vi "Text control 2 v1.1.vi"() -> ()   [LabVIEW 2016]
panel:
  in  "Serial Settings:Serial End Mode for Reads":u16(ring)=2 items=["None", "LastBit", "TermChar"]
  in  "Pump No":string="1"
  in  "bytes to read":u32=5
  in  "Timeout (ms)":u32=10000
  in  "Enable Termination\nChar (T)":bool=TRUE
  in  "Termination char\n(0xA = '\\n' = LF)\n(0xD = '\\r' = CR)":u8=13 format="%.0x"
  in  "flow control":u16(ring) items=["None"=0, "XON/XOFF"=1, "RTS/CTS"=2, "DTR/DSR"=4]
  in  "stop bits":u16(ring)=10 items=["1.0"=10, "1.5"=15, "2.0"=20]
  in  "parity":u16(ring) items=["None", "Odd", "Even", "Mark", "Space"]
  in  "data bits":u16=8 min=5 max=8 step=1
  in  "VISA resource name":refnum<visa-resource-name>="COM8"
  in  "baud rate":u32=9600
  out "Serial output":string
  out "error out":errorcluster
  in  "Units":bool
  out "Elapsed Time":dbl caption="Elapsed Time (s)"
  out "Ion vs time":cluster{"Y data in":dbl[], "X data in":dbl[]}[](graph)
  out "Ig":dbl format="%.2e"
  out "Id":dbl format="%.2e"
  out "Is":dbl format="%.2e"
  out "I vs Vg":cluster{"Y data in":dbl[], "X data in":dbl[]}[](graph)
  in  "Panel Controls 2":T1={"Emergency Stop"=refnum, "TransGraph Max"=1e-05, "Text/Graph (text=false)"=TRUE, "TransGraph Min"=1e-11} {"TransGraph Min" format="%.2e"; "TransGraph Max" format="%.2e"}
  out "Currently running:":string="#output s 0 0 0 -0.008 0.008 0.002"
  in  "Lines left to run:":string
  in  "Standby":T2
  in  "Full Reset":bool
  in  "SMU4":cluster{"on/off":bool, "Voltage":dbl} {"Voltage" min=-100.0 max=100.0 format="%.2f"}
  in  "Source/Drain Range":u8(slide)=6 max=11 scale=0.0..11.0
  in  "Source/Drain\nRange mode":u16(ring) items=["Auto", "Limited", "Fixed"]
  in  "Gate Range":u8(slide)=6 max=11 scale=0.0..11.0
  in  "Gate Range\nmode":u16(ring) items=["Auto", "Limited", "Fixed"]
  in  "Gate":T3={"Gate Start"=0.0, "Gate Stop"=2.0, "Gate Step (linear only)"=1.0, "Gate Compliance"=0.0001, "Gate PComp"=0.0, "Range mode"=0, "Range"=6} {"Range" max=11 scale=0.0..11.0; "Range mode" items=["Auto", "Limited", "Fixed"]; "Gate PComp" format="%^.2e"; "Gate Compliance" format="%^.2e"; "Gate Step (linear only)" format="%^.4e"; "Gate Stop" format="%^.4e"; "Gate Start" format="%^.4e"}
  in  "Drain 2":T4={"Drain Start"=0.0, "Drain Stop"=2.0, "Drain Compliance"=0.0001, "Drain Step"=1.0, "Drain PComp"=0.0, "Range mode"=0, "Range"=6} {"Range" max=11 scale=0.0..11.0; "Range mode" items=["Auto", "Limited", "Fixed"]; "Drain PComp" format="%^.2e"; "Drain Step" format="%^.4e"; "Drain Compliance" format="%^.2e"; "Drain Stop" format="%^.4e"; "Drain Start" format="%^.4e"}
  in  "Timings 2":T5={"integration time"=0, "Short/Long integration time"=0.00064, "hold time (sec)"=0.0, "delay time (sec)"=0.0, "Step Time (0 disables)"=0.0, "sweep method"=0, "Pulse period"=0.005, "Base voltage"=0.0, "Pulse width"=0.0005} {"Pulse width" min=0.0005 max=0.1 step=0.0001 format="%.4f"; "Base voltage" format="%^.4e"; "Pulse period" min=0.005 max=1.0 step=0.0001 format="%.4f"; "sweep method" items=["Continuous", "Pulsed"]; "Step Time (0 disables)" format="%.2f"; "delay time (sec)" format="%.4f"; "hold time (sec)" format="%.4f"; "Short/Long integration time" format="%^.0e"; "integration time" scale=0.0..2.0}
  in  "Panel Controls":T6={"Emergency Stop"=refnum, "TransGraph Max"=1e-05, "Text/Graph (text=false)"=TRUE} {"TransGraph Max" format="%.2e"}
  in  "Interrupt run":bool
  in  "Drain: Compliance":dbl=0.001 format="%.8f"
  in  "Gate: Compliance":dbl=0.001 format="%.8f"
  out "Path":path=path "C:/users/rlp38/09Apr2009LTtesting/test2.txt"
  in  "hold time /s":dbl format="%.2f"
  in  "delay time /s":dbl format="%.2f"
  in  "integration time":u32(slide) max=2 step=1 scale=0.0..2.0
  in  "Integration time (short)":dbl=0.0019 min=8e-05 max=0.0019 step=8e-05 format="%^.0e"
  in  "Integration time (long)":dbl=0.32 min=0.04 max=2.0 step=0.02 format="%.2f"
  in  "Step delay /s":dbl format="%.2f"
  in  "Program":string="#pulsedstressV d 0.03 20 0 0.5 0.0827 5\n#\n#itime s\n#gaterangemode l\n#drainrangemode l\n#pulsed on 0.05 0 0.02\n#transfer d 1 -1 -0.1 -1 -1 0\n#wait-min 1\n#transfer d 1 -1 -0.1 -1 -1 0\n#output d 0 -1 -0.5 0 -1 -0.1\n#transfer d -10 40 1 5 40 35\n#transfer d -10 40 1 5 40 35\n#output d 0 40 20 0 40 1\n#\n#\n#sample 1 0.008 221 6 0.003\n#samplei 400e-6 200 6 0.002 0.1\n#vsu2pulse -10 4\n#\n#stressV 0.016 0.03 2e-4 0.1e-3 11\n#stressI 220e-7 0.08 15\n#transfer s -1 1 0.5 -0.005 0.005 0.005\n#output s 0 0 0 -0.008 0.008 0.002\n"
  # "Syntax:\nitime [s|m|l]\ngaterangemode [a|l|f]\ndrainrangemode [a|l|f]\npulsed [on|off] PulsePeriod(sec) PulseBaseVoltage PulseONWidth(sec)\nstandby [on l off]\nwait NumMilliseconds\nwait-min NumMinutes\n# texthere = comment\ntransfer [s|d] VgStart VgStop VgStep VdStart VdStop VdStep\noutput [s|d] VgStart VgStop VgStep VdStart VdStop VdStep\nsample Vg Vd NumSamples Time(s) SampleInterval(s)\nsamplei Idg NumSamples Time(s) SampleInterval(s) VDGcompliance\n# if in doubt use SampleInterval(s) = 0.004\nstressV VG VD IGcompliance IDcompliance Duration(sec)\nstressI IDG VDGcompliance Duration(sec)\nvsu2pulse Bias Duration(s)\npulsedstressV [s|d] VEstop VgON VgOFF Period(s) PulseONwidth(s) Vd\nsample-fpp Vg Vd NumSamples Time\nresample-fpp Vg Vd\ntransfer-fpp [s|d] VgStart VgStop VgStep VdStart VdStop VdStep\noutput-fpp [s|d] VgStart VgStop VgStep VdStart VdStop VdStep"
  # "Time"
  # "Sec"
  # "Min"
  # "100 samples is approx 13s with medium integration"
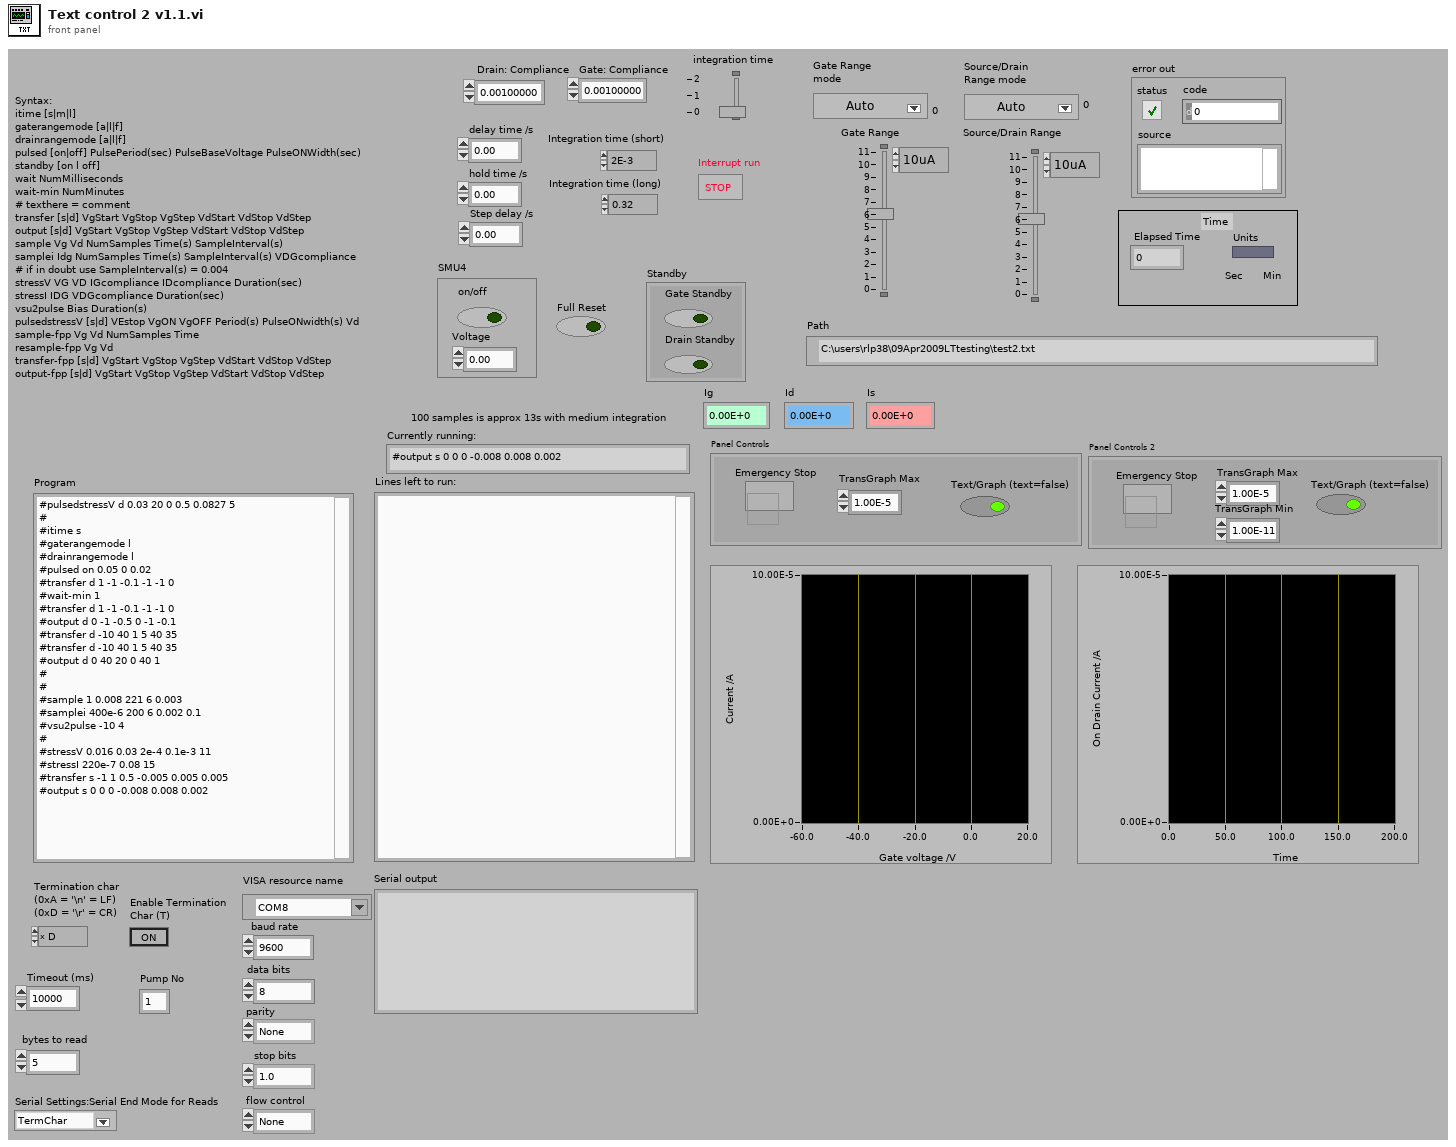
[diagram p1: front panel]
types:
  T1 = cluster{"Emergency Stop":refnum<vi>, "TransGraph Max":dbl, "Text/Graph (text=false)":bool, "TransGraph Min":dbl}
  T2 = cluster{"Gate Standby":bool, "Drain Standby":bool}
  T3 = cluster{"Gate Start":dbl, "Gate Stop":dbl, "Gate Step (linear only)":dbl, "Gate Compliance":dbl, "Gate PComp":dbl, "Range mode":u16, "Range":u8}
  T4 = cluster{"Drain Start":dbl, "Drain Stop":dbl, "Drain Compliance":dbl, "Drain Step":dbl, "Drain PComp":dbl, "Range mode":u16, "Range":u8}
  T5 = cluster{"integration time":u32, "Short/Long integration time":dbl, "hold time (sec)":dbl, "delay time (sec)":dbl, "Step Time (0 disables)":dbl, "sweep method":u16, "Pulse period":dbl, "Base voltage":dbl, "Pulse width":dbl}
  T6 = cluster{"Emergency Stop":refnum<vi>, "TransGraph Max":dbl, "Text/Graph (text=false)":bool}
  T7 = enum16{"open", "replace", "create", "open or create", "replace or create", "replace or create with confirmation"}
  T8 = cluster{"V2 Start":dbl, "V2 Step":dbl, "Number of points":i32}
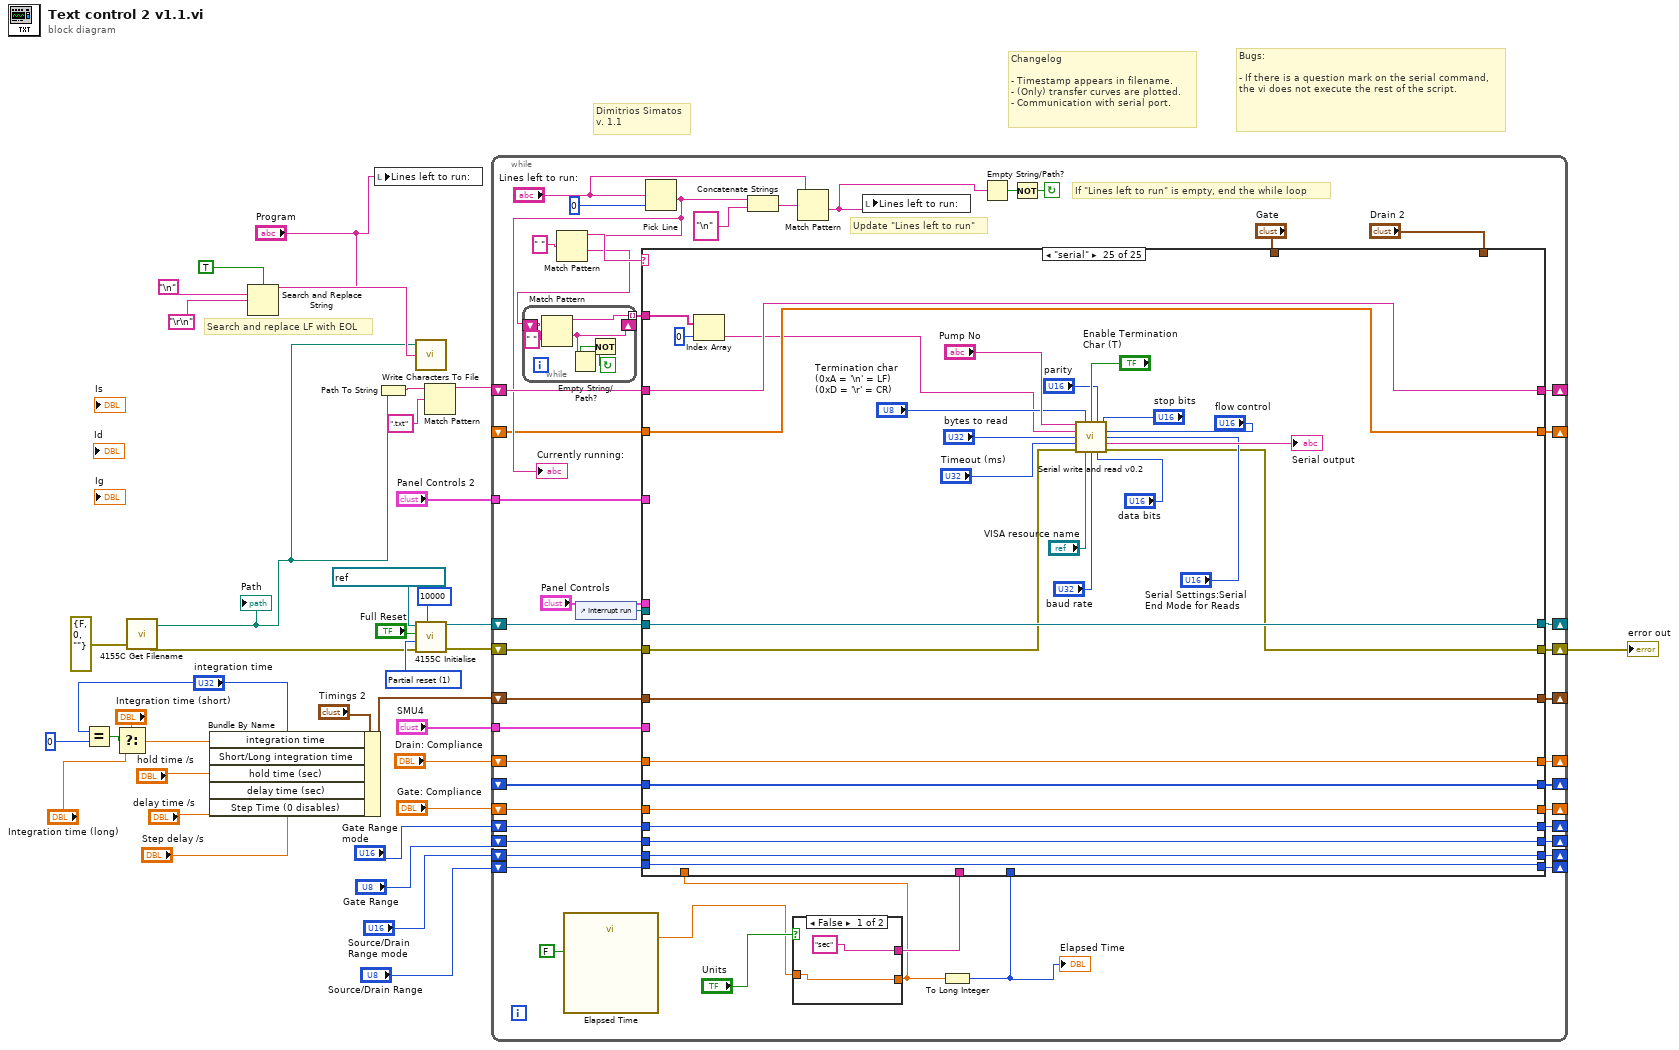
[diagram p0: block diagram]
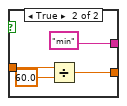
[diagram p2: hidden frame]
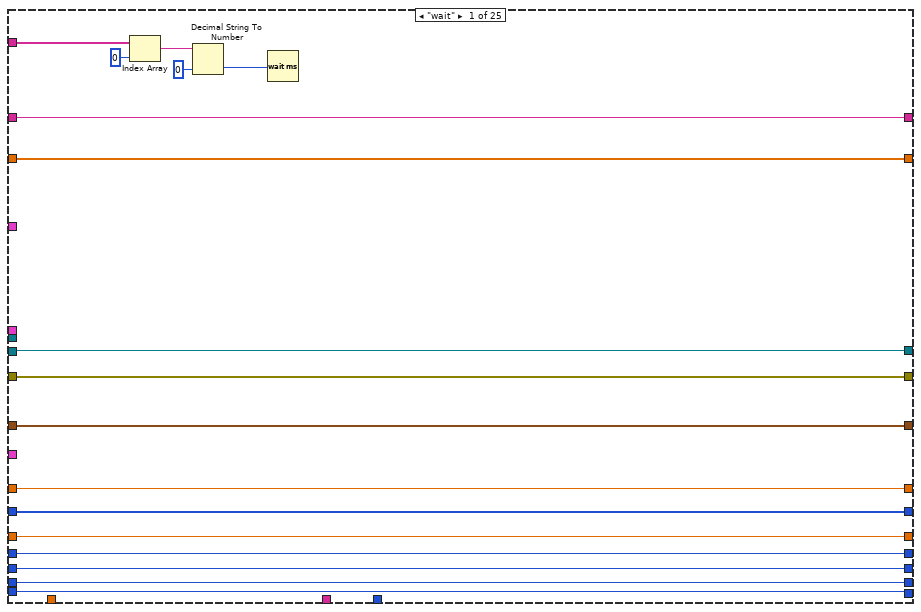
[diagram p3: hidden frame]
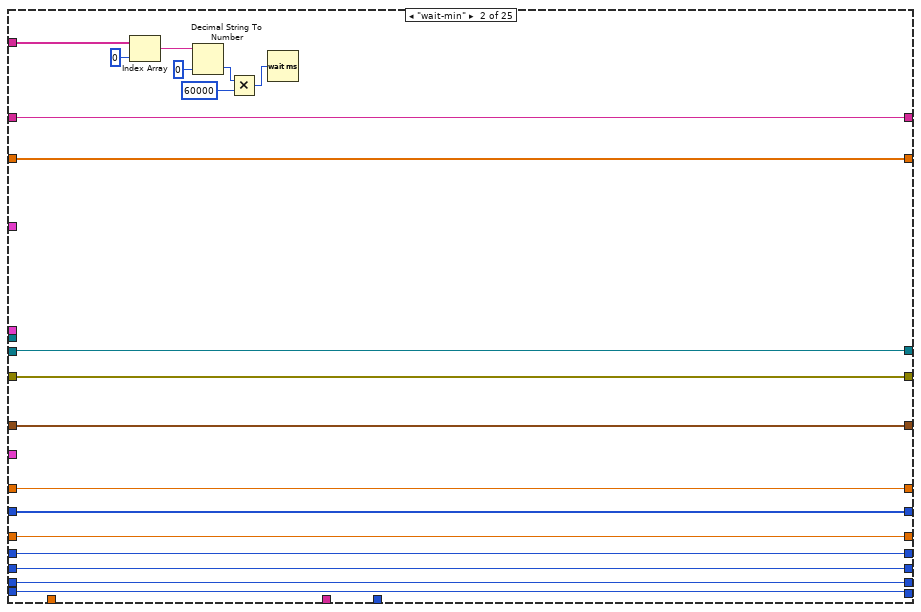
[diagram p4: hidden frame]
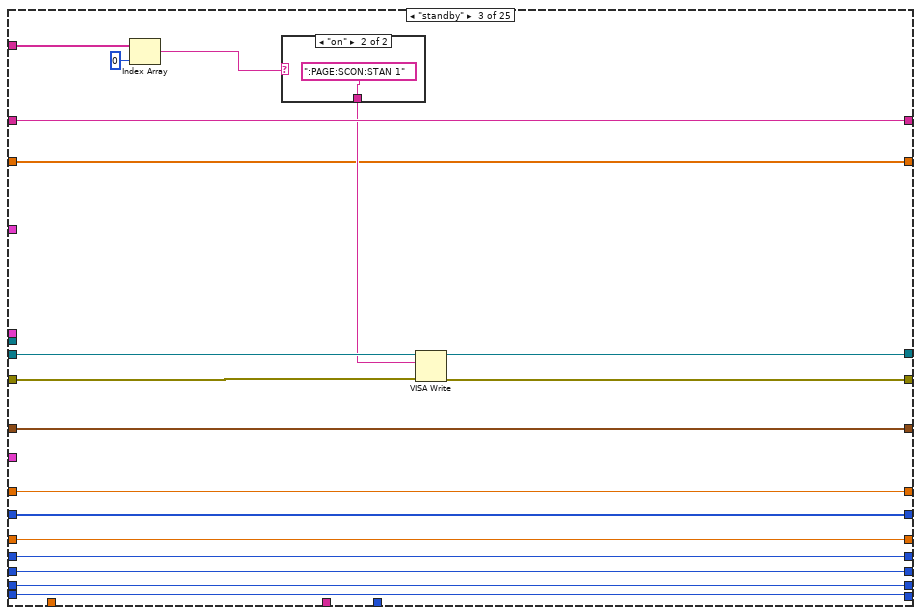
[diagram p5: hidden frame]
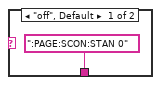
[diagram p6: hidden frame]
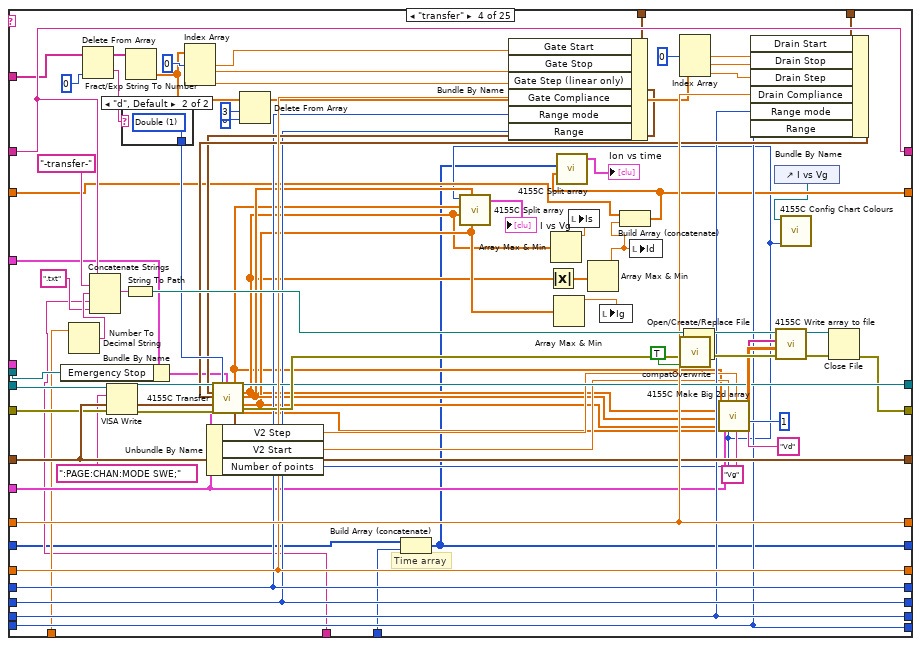
[diagram p7: hidden frame]
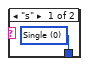
[diagram p8: hidden frame]
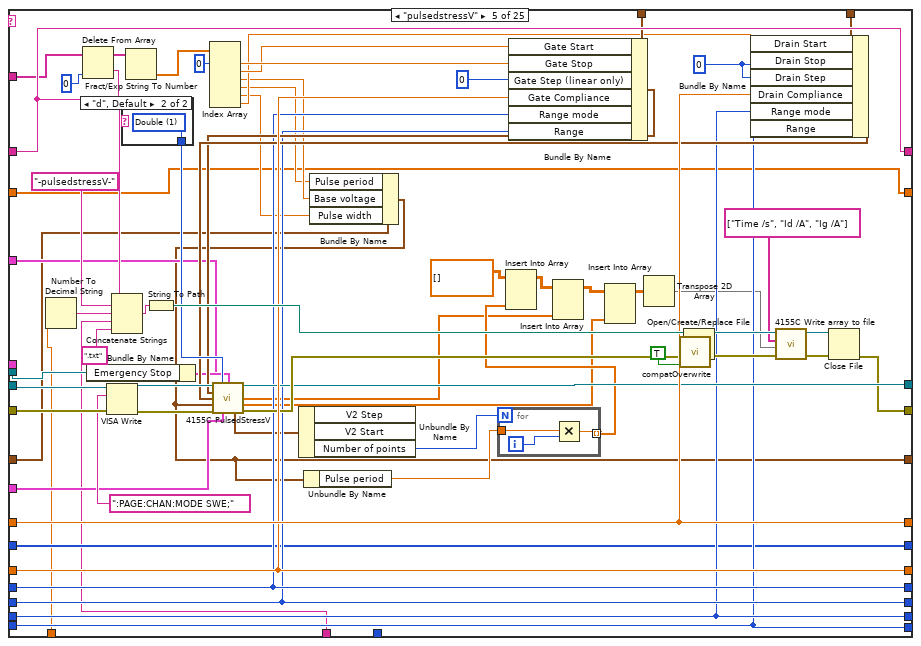
[diagram p9: hidden frame]
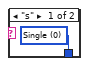
[diagram p10: hidden frame]
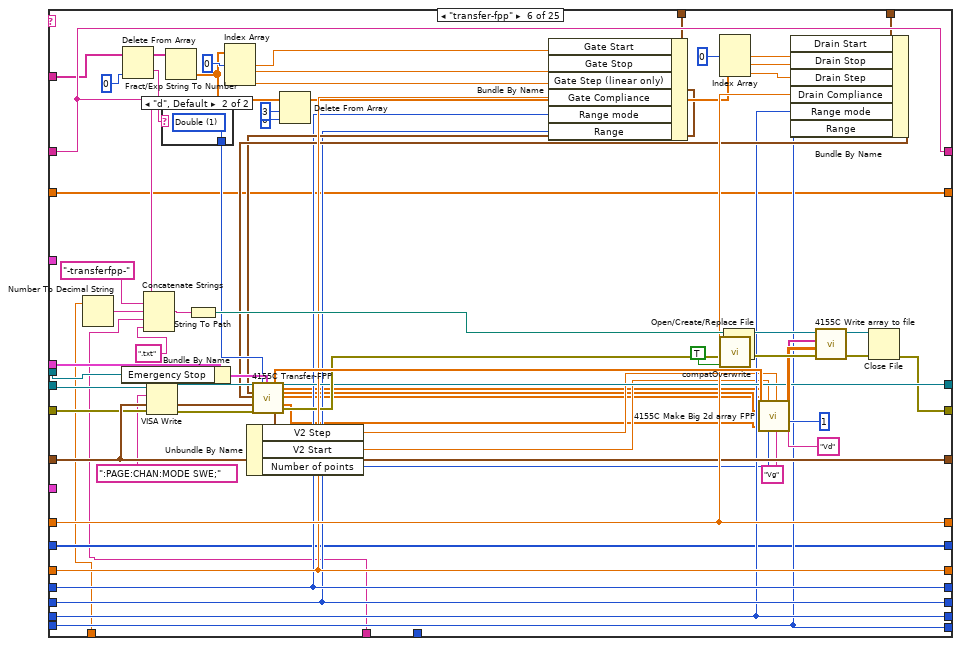
[diagram p11: hidden frame]
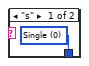
[diagram p12: hidden frame]
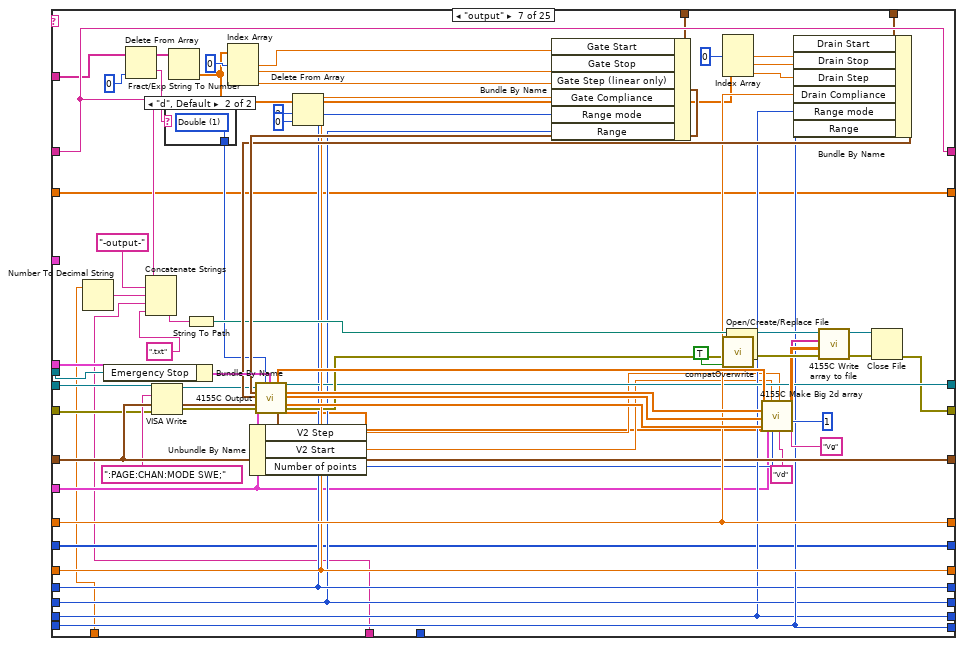
[diagram p13: hidden frame]
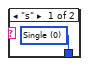
[diagram p14: hidden frame]
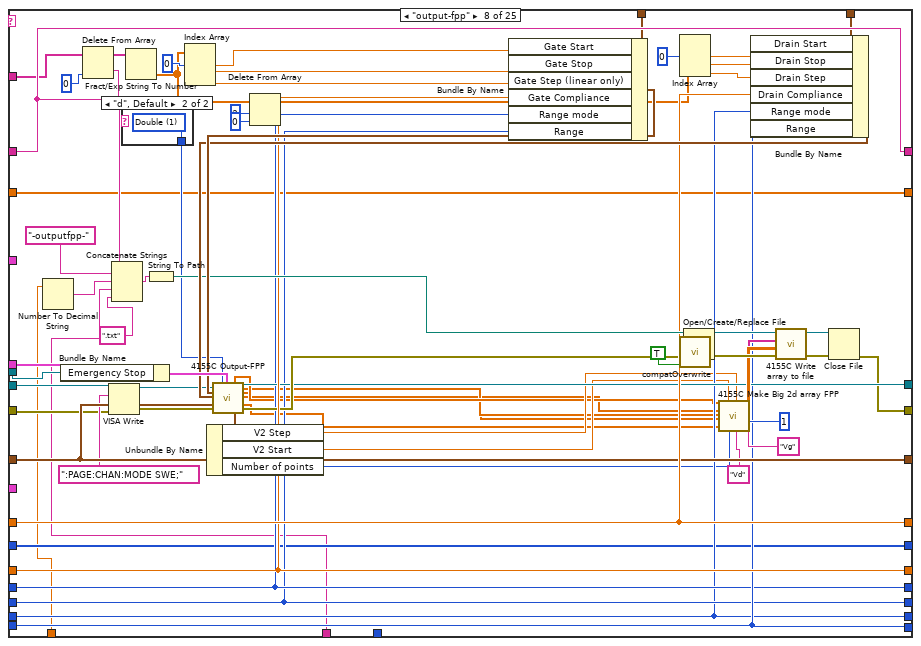
[diagram p15: hidden frame]
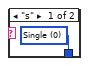
[diagram p16: hidden frame]
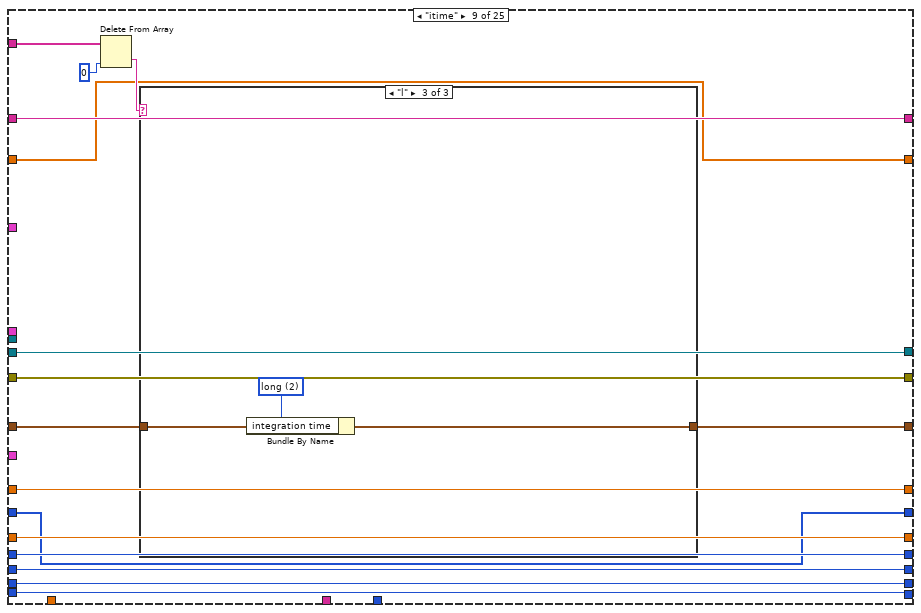
[diagram p17: hidden frame]
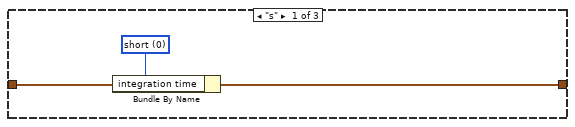
[diagram p18: hidden frame]
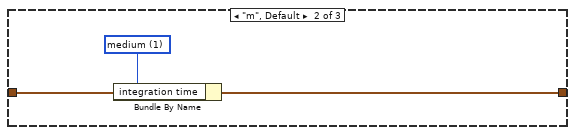
[diagram p19: hidden frame]
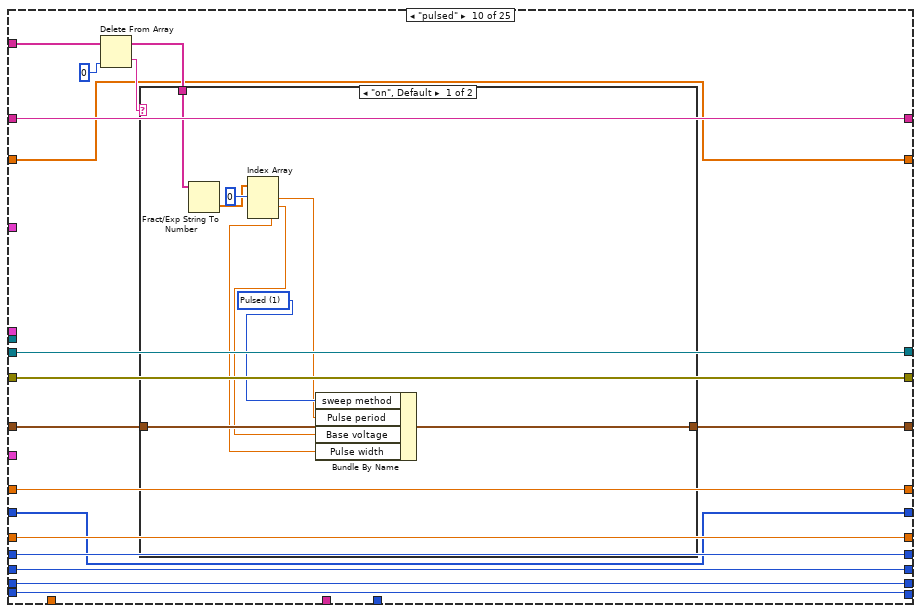
[diagram p20: hidden frame]
diagram:
  w28 = u16 1 items=["Reset All", "Partial reset"] ("Type of reset")
  # "Search and replace LF with EOL"
  # "Bugs:\n\n- If there is a question mark on the serial command, the vi does not execute the rest of the script."
  # "Dimitrios Simatos\nv. 1.1"
  # "Changelog\n\n- Timestamp appears in filename.\n- (Only) transfer curves are plotted.\n- Communication with serial port."
  n1 = Equal?(x="integration time", y=u32 0) -> (x = y?=w32:bool)
  n2 = Select(t="Integration time (short)", s=w32, f="Integration time (long)") -> (s? t:f=w36:dbl)
  n3 = call <userlib>:"4155C Get Filename.vi"("error in (no error)"=errorcluster {"status"=FALSE, "code"=0, "source"=""}) -> ("error out"=w23:errorcluster, "path"=w7:path)  [unwired: 2 in, 1 out]
  "Path" <- w7
  n4 = Bundle By Name(cluster="Timings 2", "integration time"="integration time", "Short/Long integration time"=w36, "hold time (sec)"="hold time /s", "delay time (sec)"="delay time /s", "Step Time (0 disables)"="Step delay /s") -> (w20:T5)
  n5 = Search and Replace String(replace all?=TRUE ("replace all? (F)"), input string="Program", search string="\n", replace string="\r\n") -> (result string=w10:string)  [unwired: 4 in, 3 out]
  n6 = local write "Lines left to run:"("Program") -> ()
  n7 = Path To String(path=w7) -> (string=w6:string)
  n8 = call <vilib>:"Write Characters To File.vi"("character string"=w10, "file path (dialog if empty)"=w7) -> ()  [unwired: 3 in, 1 out]
  n9 = call <userlib>:"4155C Initialise.vi"("VISA resource name in"=refnum<visa-resource-name> "GPIB0::14::INSTR", "Reset"="Full Reset", "Type of reset"=w28, "error in (no error)"=w23, "VISA Timeout Value"=u32 10000) -> ("VISA Resource Name out"=w22:refnum<visa-resource-name>, "error out"=w21:errorcluster)
  n10 = Match Pattern(string=w6, regular expression=".txt") -> (before substring=w5:string)  [unwired: 1 in, 3 out]
  n11 = while {
    tunnel: "SMU4" -> [w52]
    shift-left: "Source/Drain Range" -> [w57]
    shift-right: [w53] -> _
    shift-left: "Source/Drain\nRange mode" -> [w58]
    shift-right: [w54] -> _
    shift-left: "Gate Range" -> [w59]
    shift-right: [w55] -> _
    shift-left: "Gate Range\nmode" -> [w60]
    shift-right: [w56] -> _
    shift-left: "Gate: Compliance" -> [w71]
    shift-right: [w66] -> _
    shift-left: "Drain: Compliance" -> [w72]
    shift-right: [w67] -> _
    shift-left: w20 -> [w73]
    shift-right: [w68] -> _
    shift-left: w21 -> [w74]
    shift-right: [w69] -> w2
    shift-left: w22 -> [w75]
    shift-right: [w70] -> _
    shift-left: w5 -> [w76]
    shift-right: [w65] -> _
    tunnel: "Panel Controls 2" -> [w48]
    shift-right: [w47] -> _
    shift-left: _ -> [w46]
    shift-right: [w41] -> _
    shift-left: _ -> [w40]
    stop <- w84 continue-if-true
    # "If \"Lines left to run\" is empty, end the while loop"
    # "Update \"Lines left to run\""
    n12 = call "Elapsed Time"("Auto Reset"=FALSE) -> ("Elapsed Time (s)"=w42:dbl)  [unwired: 11 in, 7 out]
    n13 = control-ref of="Interrupt run"() -> (w64:refnum<vi>)
    n14 = Pick Line(multi-line string="Lines left to run:", line index=0) -> (output string=w49:string)  [unwired: 1 in]
    "Currently running:" <- w49
    n15 = Match Pattern(string=w49, regular expression=" ") -> (before substring=w79:string, after substring=w78:string)  [unwired: 1 in, 2 out]
    n16 = while {
      tunnel: [w92] -> w77 mode=indexing
      shift-left: w78 -> [w94]
      shift-right: [w93] -> _
      stop <- w96 continue-if-true
      n17 = Match Pattern(string=w94, regular expression=" ") -> (before substring=w92:string, after substring=w93:string)  [unwired: 1 in, 2 out]
      n18 = Empty String/Path?(string/path=w93) -> (empty?=w97:bool)
      n19 = Not(x=w97) -> (.not. x?=w96:bool)
    }
    n20 = Concatenate Strings(w49, "\n" ("Substring")) -> (w82:string)
    n21 = case shown="False" "Units" {
      tunnel: ["sec" "min"] -> w43
      tunnel: [w86 w90] -> w39
      tunnel: w42 -> [w86 w89]
      frame False {
      }
      frame True {
        n22 = Divide(x=w89, y=60.0) -> (x/y=w90:dbl)
      }
    }
    n23 = Match Pattern(string="Lines left to run:", regular expression=w82) -> (after substring=w50:string)  [unwired: 1 in, 3 out]
    n24 = local write "Lines left to run:"(w50) -> ()
    n25 = To Long Integer(number=w39) -> (32bit integer=w38:i32)
    "Elapsed Time" <- w38
    n26 = case shown="\"serial\"" w79 {
      tunnel: w77 -> [w114 w133 w151 w215 w286 w355 w422 w497 w535 w561 w588 w613 w634 w648 _ _ w752 w813 _ w878 w922 w964 w1034 w1096 w1102]
      tunnel: w76 -> [w109 w129 w149 w223 w293 w363 w430 w505 w524 w550 w580 w606 w628 w641 w660 w702 w730 w795 w826 w865 w909 w952 w1028 w1092 w1104]
      tunnel: w75 -> [w108 w128 w140 w193 w277 w332 w398 w473 w525 w551 w581 w607 w629 w642 w665 w704 w758 w819 w830 w884 w928 w970 w1040 w1050 w1108]
      tunnel: w74 -> [w107 w127 w139 w192 w276 w331 w395 w470 w526 w552 w582 w608 w630 w643 w664 w675 w757 w818 w829 w883 w927 w969 w1039 w1049 w1107]
      tunnel: w73 -> [w106 w126 w148 w219 w252 w359 w426 w501 w534 w560 w579 w605 w627 w640 w663 w699 w721 w787 w835 w858 w902 w945 w1027 w1091 w1109]
      tunnel: w72 -> [w105 w125 w147 w221 w291 w361 w428 w503 w533 w559 w587 w612 w633 w647 w662 w684 w756 w817 w838 w882 w926 w968 w1038 w1100 w1110]
      tunnel: w71 -> [w104 w124 w146 w220 w290 w360 w427 w502 w532 w558 w586 w611 w632 w646 w661 w685 w731 w796 w837 w866 w910 w953 w1029 w1093 w1112]
      tunnel: [w108 w128 w138 w217 w288 w357 w424 w499 w525 w551 w581 w607 w629 w642 w665 w704 w722 w769 w828 w859 w903 w946 w980 w1052 w1108] -> w70
      tunnel: [w107 w127 w137 w216 w287 w356 w423 w498 w526 w552 w582 w608 w630 w643 w664 w674 w732 w770 w827 w867 w911 w954 w979 w1051 w1106] -> w69
      tunnel: [w106 w126 w148 w219 w248 w359 w426 w501 w527 w553 w579 w605 w627 w640 w663 w699 w721 w787 w835 w858 w902 w945 w1027 w1091 w1109] -> w68
      tunnel: [w105 w125 w147 w221 w291 w361 w428 w503 w533 w559 w587 w612 w633 w647 w662 w684 w756 w817 w838 w882 w926 w968 w1038 w1100 w1110] -> w67
      tunnel: [w104 w124 w146 w220 w290 w360 w427 w502 w532 w558 w586 w611 w632 w646 w661 w685 w731 w796 w837 w866 w910 w953 w1029 w1093 w1112] -> w66
      tunnel: [w109 w129 w149 w223 w293 w363 w430 w505 w524 w550 w580 w606 w628 w641 w660 w702 w730 w795 w826 w865 w909 w952 w1028 w1092 w1104] -> w65
      tunnel: w64 -> [_ _ _ w226 w297 w368 w438 w509 _ _ _ _ _ _ _ _ w727 w792 _ w864 w908 w951 w1000 w1068 _]
      tunnel: "Gate" -> [_ _ _ w202 w280 w342 w409 w484 _ _ _ _ _ _ _ _ _ _ _ _ _ _ _ _ _]
      tunnel: "Drain 2" -> [_ _ _ w201 w279 w341 w408 w483 _ _ _ _ _ _ _ _ _ _ _ _ _ _ _ _ _]
      tunnel: "Panel Controls" -> [_ _ _ _ _ w340 w407 w482 _ _ _ _ _ _ _ _ _ _ _ _ _ _ _ _ _]
      tunnel: w60 -> [w103 w123 w145 w186 w270 w325 w393 w468 w531 w557 _ w604 w626 w639 w659 w686 w717 w783 w831 w854 w898 w941 w1023 w1087 w1113]
      tunnel: w59 -> [w102 w122 w144 w185 w269 w324 w392 w467 w530 w556 w585 _ w617 w645 w658 w687 w718 w784 w832 w855 w899 w942 w1024 w1088 w1114]
      tunnel: w58 -> [w101 w121 w143 w184 w268 w323 w391 w466 w529 w555 w584 w610 w631 _ w657 w688 w719 w785 w833 w856 w900 w943 w1025 w1089 w1115]
      tunnel: w57 -> [w100 w120 w142 w183 w267 w322 w394 w469 w528 w554 w583 w609 _ w644 w656 w689 w720 w786 w834 w857 w901 w944 w1026 w1090 w1116]
      tunnel: [w103 w123 w145 w186 w270 w325 w393 w468 w531 w557 w578 w604 w626 w639 w659 w686 w717 w783 w831 w854 w898 w941 w1023 w1087 w1113] -> w56
      tunnel: [w102 w122 w144 w185 w269 w324 w392 w467 w530 w556 w585 w596 w617 w645 w658 w687 w718 w784 w832 w855 w899 w942 w1024 w1088 w1114] -> w55
      tunnel: [w101 w121 w143 w184 w268 w323 w391 w466 w529 w555 w584 w610 w631 w638 w657 w688 w719 w785 w833 w856 w900 w943 w1025 w1089 w1115] -> w54
      tunnel: [w100 w120 w142 w183 w267 w322 w394 w469 w528 w554 w583 w609 w618 w644 w656 w689 w720 w786 w834 w857 w901 w944 w1026 w1090 w1116] -> w53
      tunnel: w52 -> [_ _ _ w178 w264 _ w386 _ _ _ _ _ _ _ _ _ _ _ _ _ _ _ _ _ _]
      tunnel: w48 -> [_ _ _ w176 w263 _ _ _ _ _ _ _ _ _ _ _ _ _ _ _ _ _ _ _ _]
      tunnel: [w99 w116 w135 w165 w240 w312 w383 w455 w523 w548 w577 w595 w616 w637 w655 w670 w709 w767 w825 w843 w891 w935 w977 w1045 w1105] -> w47
      tunnel: w46 -> [w99 w116 w135 w164 w240 w312 w383 w455 w523 w548 w577 w595 w616 w637 w655 w670 w709 w767 w825 w843 w891 w935 w977 w1045 w1105]
      tunnel: w39 -> [_ _ _ w160 w237 w310 w380 w452 _ _ _ _ _ _ _ w668 w707 w764 _ w840 w888 w932 w974 w1041 _]
      tunnel: w43 -> [_ _ _ w157 w236 w308 w379 w451 _ _ _ _ _ _ _ w666 w705 w763 _ w839 w887 w931 w973 w1042 _]
      tunnel: w38 -> [_ _ _ w154 _ _ _ _ _ _ _ _ _ _ _ _ _ _ _ _ _ _ _ _ _]
      tunnel: [w98 w115 w134 w156 w239 w311 w382 w454 w522 w547 w576 w594 w615 w636 w654 w669 w708 w766 w824 w842 w890 w934 w976 w1044 w1111] -> w41
      tunnel: w40 -> [w98 w115 w134 w155 w239 w311 w382 w454 w522 w547 w576 w594 w615 w636 w654 w669 w708 w766 w824 w842 w890 w934 w976 w1044 w1111]
      frame "wait" {
        n27 = Index Array(array=w114, index=0 ("Index")) -> (element=w112:string)
        n28 = Decimal String To Number(string=w112, default (0L)=u32 0) -> (number=w111:u32)  [unwired: 1 in, 1 out]
        n29 = Wait (ms)(milliseconds to wait=w111) -> ()  [unwired: 1 out]
      }
      frame "wait-min" {
        n30 = Index Array(array=w133, index=0 ("Index")) -> (element=w131:string)
        n31 = Decimal String To Number(string=w131, default (0L)=u32 0) -> (number=w119:u32)  [unwired: 1 in, 1 out]
        n32 = Multiply(x=w119, y=u32 60000) -> (x*y=w118:u32)
        n33 = Wait (ms)(milliseconds to wait=w118) -> ()  [unwired: 1 out]
      }
      frame "standby" {
        n34 = Index Array(array=w151, index=0 ("Index")) -> (element=w141:string)
        n35 = case shown="\"on\"" w141 {
          tunnel: [":PAGE:SCON:STAN 0" ":PAGE:SCON:STAN 1"] -> w136
          frame "off", Default {
          }
          frame "on" {
          }
        }
        n36 = VISA Write(VISA resource name=w140, write buffer=w136, error in (no error)=w139) -> (VISA resource name out=w138:refnum<visa-resource-name>, error out=w137:errorcluster)  [unwired: 1 out]
      }
      frame "transfer" {
        # "Time array"
        n37 = Bundle By Name(cluster=w176, "Emergency Stop"=w226) -> (w177:T1)
        n38 = Number To Decimal String(number=w160) -> (decimal integer string=w159:string)  [unwired: 1 in]
        n39 = Delete From Array(array=w215, index=0 ("Index")) -> (deleted portion=w213:string, array with subset deleted=w212:string[])  [unwired: 1 in]
        n40 = Concatenate Strings(w223, "-transfer-" ("Prefix"), w159, w157, ".txt" ("Suffix")) -> (w225:string)
        n41 = VISA Write(VISA resource name=w193, write buffer=":PAGE:CHAN:MODE SWE;" ("write buffer (\"\")"), error in (no error)=w192) -> (VISA resource name out=w190:refnum<visa-resource-name>, error out=w191:errorcluster)  [unwired: 1 out]
        n42 = case shown="\"d\", Default" w213 {
          tunnel: [w234 w235] -> w211
          frame "s" {
            w234 = u16 0 items=["Single", "Double"] ("sweep mode")
          }
          frame "d", Default {
            w235 = u16 1 items=["Single", "Double"] ("sweep mode")
          }
        }
        n43 = String To Path(string=w225) -> (path=w222:path)
        n44 = Fract/Exp String To Number(string=w212) -> (number=w197:dbl[])  [unwired: 3 in, 1 out]
        n45 = Index Array(array=w197, index #1=0 ("Index")) -> (element #1=w210:dbl, element #2=w209:dbl, element #3=w208:dbl)  [unwired: 2 in]
        n46 = Delete From Array(array=w197, length=3 ("Length"), index=0 ("Index")) -> (array with subset deleted=w195:dbl[])  [unwired: 1 out]
        n47 = Build Array (concatenate)(w155, w154) -> (w156:i32[])
        n48 = Bundle By Name(cluster=w202, "Gate Start"=w210, "Gate Stop"=w209, "Gate Step (linear only)"=w208, "Gate Compliance"=w220, "Range mode"=w186, "Range"=w185) -> (w187:T3)
        n49 = Index Array(array=w195, index #1=0 ("Index")) -> (element #1=w205:dbl, element #2=w204:dbl, element #3=w203:dbl)  [unwired: 2 in]
        n50 = call <vilib>:"compatOverwrite.vi"("overwrite (F)"=TRUE) -> ("overwrite?"=w175:T7)
        n51 = Bundle By Name(cluster=w201, "Drain Start"=w205, "Drain Stop"=w204, "Drain Step"=w203, "Drain Compliance"=w221, "Range mode"=w184, "Range"=w183) -> (w188:T4)
        n52 = call <userlib>:"4155C Transfer.vi"("VISA resource name in"=w190, "Gate"=w187, "Drain"=w188, "Timings"=w219, "error in (no error)"=w191, "SMU4"=w178, "sweep mode"=w211, "Panel Controls"=w177) -> ("VG"=w166:dbl[], "Outparams"=w182:T8, "VISA Resource Name out"=w217:refnum<visa-resource-name>, "IS"=w168:dbl[], "ID"=w173:dbl[], "IG"=w169:dbl[], "error out"=w218:errorcluster, "SMU4"=w179:dbl[])  [unwired: 12 in]
        n53 = Unbundle By Name(w182) -> ("V2 Step"=w181:dbl, "V2 Start"=w180:dbl, "Number of points"=w162:i32)
        n54 = call <userlib>:"4155C Split array.vi"("Number of VAR2 steps"=w162, "Y2 data in"=w173, "X data in"=w166, "Y1 data in"=w168, "Y3 data in"=w169) -> ("Array of clusters"=→"I vs Vg":cluster{"Y data in":dbl[], "X data in":dbl[]}[])  [unwired: 2 in, 1 out]
        n55 = Absolute Value(x=w168) -> (abs(x)=w172:dbl[])
        n56 = Array Max & Min(array=w168) -> (max value=w170:dbl)  [unwired: 3 out]
        n57 = Array Max & Min(array=w169) -> (max value=w171:dbl)  [unwired: 3 out]
        n58 = local write "Is"(w170) -> ()
        n59 = Array Max & Min(array=w172) -> (max value=w163:dbl)  [unwired: 3 out]
        n60 = local write "Ig"(w171) -> ()
        n61 = Build Array (concatenate)(w164, w163) -> (w165:dbl[])
        n62 = call <userlib>:"4155C Split array.vi"("X data in"=w156, "Y1 data in"=w165) -> ("Array of clusters"=→"Ion vs time":cluster{"Y data in":dbl[], "X data in":dbl[]}[])  [unwired: 5 in, 1 out]
        n63 = local write "Id"(w163) -> ()
        n64 = Open/Create/Replace File(file path (use dialog)=w222, error in=w218, operation (0:open)=w175) -> (refnum out=w231:refnum<file>, error out=w232:errorcluster)  [unwired: 3 in, 1 out]
        n65 = call <userlib>:"4155C Make Big 2d array.vi"("1D Var1"=w166, "1d IS"=w168, "1d ID"=w173, "1d IG"=w169, "1d SMU4"=w179, "SMU4"=w178, "VAR2 START"=w180, "Number of VAR2 steps"=w162, "VAR2 STEP"=w181, "VAR1 Name"="Vg", "Decimal places in header"=i8 1, "VAR2 Name"="Vd") -> ("Header array"=w227:string[], "Data array"=w228:dbl[][])  [unwired: 14 in]
        n66 = control-ref of="I vs Vg"() -> (w161:refnum<vi>)
        n67 = call <userlib>:"4155C Write array to file.vi"("Byte Stream File Refnum"=w231, "Header"=w227, "Data Array"=w228, "error in (no error)"=w232) -> ("dup refnum"=w229:refnum<file>, "error out"=w230:errorcluster)  [unwired: 1 in]
        n68 = call <userlib>:"4155C Config Chart Colours.vi"("Numeric"=w162, "XY Graph 2"=w161) -> ()  [unwired: 6 in]
        n69 = Close File(refnum=w229, error in=w230) -> (error out=w216:errorcluster)  [unwired: 1 out]
      }
      frame "pulsedstressV" {
        w246 = 0
        n70 = Number To Decimal String(number=w237) -> (decimal integer string=w294:string)  [unwired: 1 in]
        n71 = Delete From Array(array=w286, index=0 ("Index")) -> (deleted portion=w284:string, array with subset deleted=w283:string[])  [unwired: 1 in]
        n72 = Bundle By Name(cluster=w263, "Emergency Stop"=w297) -> (w265:T1)
        n73 = VISA Write(VISA resource name=w277, write buffer=":PAGE:CHAN:MODE SWE;" ("write buffer (\"\")"), error in (no error)=w276) -> (VISA resource name out=w274:refnum<visa-resource-name>, error out=w275:errorcluster)  [unwired: 1 out]
        n74 = Concatenate Strings(w293, "-pulsedstressV-" ("Substring"), w294, w236, ".txt" ("Substring")) -> (w296:string)
        n75 = case shown="\"d\", Default" w284 {
          tunnel: [w306 w307] -> w282
          frame "s" {
            w306 = u16 0 items=["Single", "Double"] ("sweep mode")
          }
          frame "d", Default {
            w307 = u16 1 items=["Single", "Double"] ("sweep mode")
          }
        }
        n76 = Fract/Exp String To Number(string=w283) -> (number=w278:dbl[])  [unwired: 3 in, 1 out]
        n77 = String To Path(string=w296) -> (path=w292:path)
        n78 = Index Array(array=w278, index #1=0 ("Index")) -> (element #1=w255:dbl, element #2=w254:dbl, element #3=w251:dbl, element #4=w250:dbl, element #5=w249:dbl, element #6=w253:dbl)  [unwired: 5 in]
        n79 = Bundle By Name(cluster=w252, "Pulse period"=w250, "Base voltage"=w251, "Pulse width"=w249) -> (w248:T5)
        n80 = Unbundle By Name(w248) -> ("Pulse period"=w256:dbl)
        n81 = Bundle By Name(cluster=w280, "Gate Start"=w254, "Gate Stop"=w255, "Gate Step (linear only)"=0, "Gate Compliance"=w290, "Range mode"=w270, "Range"=w269) -> (w271:T3)
        n82 = call <vilib>:"compatOverwrite.vi"("overwrite (F)"=TRUE) -> ("overwrite?"=w241:T7)
        n83 = Bundle By Name(cluster=w279, "Drain Start"=w253, "Drain Stop"=w246, "Drain Step"=w246, "Drain Compliance"=w291, "Range mode"=w268, "Range"=w267) -> (w272:T4)
        n84 = call <userlib>:"4155C PulsedStressV.vi"("VISA resource name in"=w274, "sweep mode"=w282, "Panel Controls"=w265, "Gate"=w271, "Drain"=w272, "Timings"=w248, "error in (no error)"=w275, "SMU4"=w264) -> ("VISA Resource Name out"=w288:refnum<visa-resource-name>, "ID"=w244:dbl[], "IG"=w242:dbl[], "Outparams"=w266:T8, "error out"=w289:errorcluster)  [unwired: 3 in]
        n85 = Unbundle By Name(w266) -> ("Number of points"=w243:i32)  [unwired: 2 out]
        n86 = for {
          N: w243 -> [_]
          tunnel: [w303] -> w245 mode=indexing
          tunnel: w256 -> [w305]
          i -> [w304]
          n87 = Multiply(x=w305, y=w304) -> (x*y=w303:dbl)
        }
        n88 = Insert Into Array(array=dbl[][] [] ("Input Array"), new element=w245) -> (w257:dbl[][])  [unwired: 2 in]
        n89 = Insert Into Array(array=w257, new element=w244) -> (w262:dbl[][])  [unwired: 2 in]
        n90 = Insert Into Array(array=w262, new element=w242) -> (w261:dbl[][])  [unwired: 2 in]
        n91 = Transpose 2D Array(2D array=w261) -> (transposed array=w260:dbl[][])
        n92 = Open/Create/Replace File(file path (use dialog)=w292, error in=w289, operation (0:open)=w241) -> (refnum out=w300:refnum<file>, error out=w301:errorcluster)  [unwired: 3 in, 1 out]
        n93 = call <userlib>:"4155C Write array to file.vi"("Byte Stream File Refnum"=w300, "Header"=string[] ["Time /s", "Id /A", "Ig /A"], "Data Array"=w260, "error in (no error)"=w301) -> ("dup refnum"=w298:refnum<file>, "error out"=w299:errorcluster)  [unwired: 1 in]
        n94 = Close File(refnum=w298, error in=w299) -> (error out=w287:errorcluster)  [unwired: 1 out]
      }
      frame "transfer-fpp" {
        n95 = Number To Decimal String(number=w310) -> (decimal integer string=w364:string)  [unwired: 1 in]
        n96 = Bundle By Name(cluster=w340, "Emergency Stop"=w368) -> (w376:T6)
        n97 = Delete From Array(array=w355, index=0 ("Index")) -> (deleted portion=w353:string, array with subset deleted=w352:string[])  [unwired: 1 in]
        n98 = Concatenate Strings(w363, "-transferfpp-" ("Substring"), w364, w308, ".txt" ("Substring")) -> (w366:string)
        n99 = VISA Write(VISA resource name=w332, write buffer=":PAGE:CHAN:MODE SWE;" ("write buffer (\"\")"), error in (no error)=w331) -> (VISA resource name out=w329:refnum<visa-resource-name>, error out=w330:errorcluster)  [unwired: 1 out]
        n100 = case shown="\"d\", Default" w353 {
          tunnel: [w377 w378] -> w351
          frame "s" {
            w377 = u16 0 items=["Single", "Double"] ("sweep mode")
          }
          frame "d", Default {
            w378 = u16 1 items=["Single", "Double"] ("sweep mode")
          }
        }
        n101 = Fract/Exp String To Number(string=w352) -> (number=w336:dbl[])  [unwired: 3 in, 1 out]
        n102 = String To Path(string=w366) -> (path=w362:path)
        n103 = Index Array(array=w336, index #1=0 ("Index")) -> (element #1=w350:dbl, element #2=w349:dbl, element #3=w348:dbl)  [unwired: 2 in]
        n104 = Delete From Array(array=w336, length=3 ("Length"), index=0 ("Index")) -> (array with subset deleted=w334:dbl[])  [unwired: 1 out]
        n105 = Bundle By Name(cluster=w342, "Gate Start"=w350, "Gate Stop"=w349, "Gate Step (linear only)"=w348, "Gate Compliance"=w360, "Range mode"=w325, "Range"=w324) -> (w326:T3)
        n106 = Index Array(array=w334, index #1=0 ("Index")) -> (element #1=w345:dbl, element #2=w344:dbl, element #3=w343:dbl)  [unwired: 2 in]
        n107 = call <vilib>:"compatOverwrite.vi"("overwrite (F)"=TRUE) -> ("overwrite?"=w313:T7)
        n108 = Bundle By Name(cluster=w341, "Drain Start"=w345, "Drain Stop"=w344, "Drain Step"=w343, "Drain Compliance"=w361, "Range mode"=w323, "Range"=w322) -> (w327:T4)
        n109 = call <userlib>:"4155C Transfer-FPP.vi"("VISA resource name in"=w329, "Gate"=w326, "Drain"=w327, "Timings"=w359, "error in (no error)"=w330, "sweep mode"=w351, "Panel Controls"=w376) -> ("VG"=w367:dbl[], "Outparams"=w321:T8, "VISA Resource Name out"=w357:refnum<visa-resource-name>, "Vprobe2"=w317:dbl[], "ID"=w316:dbl[], "IG"=w315:dbl[], "Vprobe1"=w314:dbl[], "error out"=w358:errorcluster)  [unwired: 13 in]
        n110 = Unbundle By Name(w321) -> ("V2 Step"=w320:dbl, "V2 Start"=w319:dbl, "Number of points"=w318:i32)
        n111 = Open/Create/Replace File(file path (use dialog)=w362, error in=w358, operation (0:open)=w313) -> (refnum out=w373:refnum<file>, error out=w374:errorcluster)  [unwired: 3 in, 1 out]
        n112 = call <userlib>:"4155C Make Big 2d array FPP.vi"("1D Var1"=w367, "1d ID"=w316, "1d Vp2"=w317, "1d IG"=w315, "1d Vp1"=w314, "VAR2 START"=w319, "Number of VAR2 steps"=w318, "VAR2 STEP"=w320, "VAR1 Name"="Vg", "Decimal places in header"=i8 1, "VAR2 Name"="Vd") -> ("Header array"=w369:string[], "Data array"=w370:dbl[][])  [unwired: 15 in]
        n113 = call <userlib>:"4155C Write array to file.vi"("Byte Stream File Refnum"=w373, "Header"=w369, "Data Array"=w370, "error in (no error)"=w374) -> ("dup refnum"=w371:refnum<file>, "error out"=w372:errorcluster)  [unwired: 1 in]
        n114 = Close File(refnum=w371, error in=w372) -> (error out=w356:errorcluster)  [unwired: 1 out]
      }
      frame "output" {
        n115 = Number To Decimal String(number=w380) -> (decimal integer string=w431:string)  [unwired: 1 in]
        n116 = Bundle By Name(cluster=w407, "Emergency Stop"=w438) -> (w448:T6)
        n117 = Delete From Array(array=w422, index=0 ("Index")) -> (deleted portion=w420:string, array with subset deleted=w419:string[])  [unwired: 1 in]
        n118 = Concatenate Strings(w430, "-output-" ("Substring"), w431, w379, ".txt" ("Substring")) -> (w433:string)
        n119 = VISA Write(VISA resource name=w398, write buffer=":PAGE:CHAN:MODE SWE;" ("write buffer (\"\")"), error in (no error)=w395) -> (VISA resource name out=w397:refnum<visa-resource-name>, error out=w396:errorcluster)  [unwired: 1 out]
        n120 = case shown="\"d\", Default" w420 {
          tunnel: [w449 w450] -> w418
          frame "s" {
            w449 = u16 0 items=["Single", "Double"] ("sweep mode")
          }
          frame "d", Default {
            w450 = u16 1 items=["Single", "Double"] ("sweep mode")
          }
        }
        n121 = Fract/Exp String To Number(string=w419) -> (number=w401:dbl[])  [unwired: 3 in, 1 out]
        n122 = String To Path(string=w433) -> (path=w429:path)
        n123 = Index Array(array=w401, index #1=0 ("Index")) -> (element #1=w417:dbl, element #2=w416:dbl, element #3=w415:dbl)  [unwired: 2 in]
        n124 = Delete From Array(array=w401, length=3 ("Length"), index=0 ("Index")) -> (array with subset deleted=w400:dbl[])  [unwired: 1 out]
        n125 = Bundle By Name(cluster=w409, "Gate Start"=w417, "Gate Stop"=w416, "Gate Step (linear only)"=w415, "Gate Compliance"=w427, "Range mode"=w393, "Range"=w392) -> (w447:T3)
        n126 = Index Array(array=w400, index #1=0 ("Index")) -> (element #1=w412:dbl, element #2=w411:dbl, element #3=w410:dbl)  [unwired: 2 in]
        n127 = call <vilib>:"compatOverwrite.vi"("overwrite (F)"=TRUE) -> ("overwrite?"=w384:T7)
        n128 = Bundle By Name(cluster=w408, "Drain Start"=w412, "Drain Stop"=w411, "Drain Step"=w410, "Drain Compliance"=w428, "Range mode"=w391, "Range"=w394) -> (w446:T4)
        n129 = call <userlib>:"4155C Output.vi"("VISA resource name in"=w397, "Gate"=w447, "Drain"=w446, "Timings"=w426, "error in (no error)"=w396, "SMU4"=w386, "sweep mode"=w418, "Panel controls"=w448) -> ("VD"=w434:dbl[], "Outparams"=w389:T8, "VISA Resource Name out"=w424:refnum<visa-resource-name>, "IS"=w437:dbl[], "ID"=w436:dbl[], "IG"=w435:dbl[], "error out"=w425:errorcluster, "SMU4"=w385:dbl[])  [unwired: 12 in]
        n130 = Unbundle By Name(w389) -> ("V2 Step"=w390:dbl, "V2 Start"=w388:dbl, "Number of points"=w387:i32)
        n131 = Open/Create/Replace File(file path (use dialog)=w429, error in=w425, operation (0:open)=w384) -> (refnum out=w443:refnum<file>, error out=w444:errorcluster)  [unwired: 3 in, 1 out]
        n132 = call <userlib>:"4155C Make Big 2d array.vi"("1D Var1"=w434, "1d IS"=w437, "1d ID"=w436, "1d IG"=w435, "1d SMU4"=w385, "SMU4"=w386, "VAR2 START"=w388, "Number of VAR2 steps"=w387, "VAR2 STEP"=w390, "VAR1 Name"="Vd", "Decimal places in header"=i8 1, "VAR2 Name"="Vg") -> ("Header array"=w439:string[], "Data array"=w440:dbl[][])  [unwired: 14 in]
        n133 = call <userlib>:"4155C Write array to file.vi"("Byte Stream File Refnum"=w443, "Header"=w439, "Data Array"=w440, "error in (no error)"=w444) -> ("dup refnum"=w441:refnum<file>, "error out"=w442:errorcluster)  [unwired: 1 in]
        n134 = Close File(refnum=w441, error in=w442) -> (error out=w423:errorcluster)  [unwired: 1 out]
      }
      frame "output-fpp" {
        n135 = Number To Decimal String(number=w452) -> (decimal integer string=w506:string)  [unwired: 1 in]
        n136 = Bundle By Name(cluster=w482, "Emergency Stop"=w509) -> (w519:T6)
        n137 = Delete From Array(array=w497, index=0 ("Index")) -> (deleted portion=w495:string, array with subset deleted=w494:string[])  [unwired: 1 in]
        n138 = VISA Write(VISA resource name=w473, write buffer=":PAGE:CHAN:MODE SWE;" ("write buffer (\"\")"), error in (no error)=w470) -> (VISA resource name out=w472:refnum<visa-resource-name>, error out=w471:errorcluster)  [unwired: 1 out]
        n139 = Concatenate Strings(w505, "-outputfpp-" ("Substring"), w506, w451, ".txt" ("Substring")) -> (w508:string)
        n140 = case shown="\"d\", Default" w495 {
          tunnel: [w520 w521] -> w493
          frame "s" {
            w520 = u16 0 items=["Single", "Double"] ("sweep mode")
          }
          frame "d", Default {
            w521 = u16 1 items=["Single", "Double"] ("sweep mode")
          }
        }
        n141 = Fract/Exp String To Number(string=w494) -> (number=w476:dbl[])  [unwired: 3 in, 1 out]
        n142 = String To Path(string=w508) -> (path=w504:path)
        n143 = Index Array(array=w476, index #1=0 ("Index")) -> (element #1=w492:dbl, element #2=w491:dbl, element #3=w490:dbl)  [unwired: 2 in]
        n144 = Delete From Array(array=w476, length=3 ("Length"), index=0 ("Index")) -> (array with subset deleted=w475:dbl[])  [unwired: 1 out]
        n145 = Bundle By Name(cluster=w484, "Gate Start"=w492, "Gate Stop"=w491, "Gate Step (linear only)"=w490, "Gate Compliance"=w502, "Range mode"=w468, "Range"=w467) -> (w518:T3)
        n146 = Index Array(array=w475, index #1=0 ("Index")) -> (element #1=w487:dbl, element #2=w486:dbl, element #3=w485:dbl)  [unwired: 2 in]
        n147 = call <vilib>:"compatOverwrite.vi"("overwrite (F)"=TRUE) -> ("overwrite?"=w456:T7)
        n148 = Bundle By Name(cluster=w483, "Drain Start"=w487, "Drain Stop"=w486, "Drain Step"=w485, "Drain Compliance"=w503, "Range mode"=w466, "Range"=w469) -> (w517:T4)
        n149 = call <userlib>:"4155C Output-FPP.vi"("VISA resource name in"=w472, "Gate"=w518, "Drain"=w517, "Timings"=w501, "error in (no error)"=w471, "sweep mode"=w493, "Panel controls"=w519) -> ("VD"=w461:dbl[], "Outparams"=w464:T8, "VISA Resource Name out"=w499:refnum<visa-resource-name>, "Vprobe2"=w460:dbl[], "ID"=w459:dbl[], "IG"=w458:dbl[], "Vprobe1"=w457:dbl[], "error out"=w500:errorcluster)  [unwired: 13 in]
        n150 = Unbundle By Name(w464) -> ("V2 Step"=w465:dbl, "V2 Start"=w463:dbl, "Number of points"=w462:i32)
        n151 = Open/Create/Replace File(file path (use dialog)=w504, error in=w500, operation (0:open)=w456) -> (refnum out=w514:refnum<file>, error out=w515:errorcluster)  [unwired: 3 in, 1 out]
        n152 = call <userlib>:"4155C Make Big 2d array FPP.vi"("1D Var1"=w461, "1d ID"=w459, "1d Vp2"=w460, "1d IG"=w458, "1d Vp1"=w457, "VAR2 START"=w463, "Number of VAR2 steps"=w462, "VAR2 STEP"=w465, "VAR1 Name"="Vd", "Decimal places in header"=i8 1, "VAR2 Name"="Vg") -> ("Header array"=w510:string[], "Data array"=w511:dbl[][])  [unwired: 15 in]
        n153 = call <userlib>:"4155C Write array to file.vi"("Byte Stream File Refnum"=w514, "Header"=w510, "Data Array"=w511, "error in (no error)"=w515) -> ("dup refnum"=w512:refnum<file>, "error out"=w513:errorcluster)  [unwired: 1 in]
        n154 = Close File(refnum=w512, error in=w513) -> (error out=w498:errorcluster)  [unwired: 1 out]
      }
      frame "itime" {
        n155 = Delete From Array(array=w535, index=0 ("Index")) -> (deleted portion=w536:string)  [unwired: 1 in, 1 out]
        n156 = case shown="\"l\"" w536 {
          tunnel: w534 -> [w540 w542 w545]
          tunnel: [w539 w541 w544] -> w527
          frame "s" {
            w538 = u32 0 items=["short  ", "medium  ", "long  "] ("integration time 2")
            n157 = Bundle By Name(cluster=w540, "integration time"=w538) -> (w539:T5)
          }
          frame "m", Default {
            w543 = u32 1 items=["short  ", "medium  ", "long  "] ("integration time 2")
            n158 = Bundle By Name(cluster=w542, "integration time"=w543) -> (w541:T5)
          }
          frame "l" {
            w546 = u32 2 items=["short  ", "medium  ", "long  "] ("integration time 2")
            n159 = Bundle By Name(cluster=w545, "integration time"=w546) -> (w544:T5)
          }
        }
      }
      frame "pulsed" {
        n160 = Delete From Array(array=w561, index=0 ("Index")) -> (deleted portion=w562:string, array with subset deleted=w549:string[])  [unwired: 1 in]
        n161 = case shown="\"on\", Default" w562 {
          tunnel: w560 -> [w572 w575]
          tunnel: [w571 w574] -> w553
          tunnel: w549 -> [w569 _]
          frame "on", Default {
            w570 = u16 1 items=["Continuous", "Pulsed"] ("sweep method")
            n162 = Fract/Exp String To Number(string=w569) -> (number=w567:dbl[])  [unwired: 3 in, 1 out]
            n163 = Index Array(array=w567, index #1=0 ("Index")) -> (element #1=w566:dbl, element #2=w565:dbl, element #3=w564:dbl)  [unwired: 2 in]
            n164 = Bundle By Name(cluster=w572, "sweep method"=w570, "Pulse period"=w566, "Base voltage"=w565, "Pulse width"=w564) -> (w571:T5)
          }
          frame "off" {
            w573 = u16 0 items=["Continuous", "Pulsed"] ("sweep method")
            n165 = Bundle By Name(cluster=w575, "sweep method"=w573) -> (w574:T5)
          }
        }
      }
      frame "gaterangemode" {
        n166 = Delete From Array(array=w588, index=0 ("Index")) -> (deleted portion=w589:string)  [unwired: 1 in, 1 out]
        n167 = case shown="\"f\"" w589 {
          tunnel: [w591 w592 w593] -> w578
          frame "a", Default {
            w591 = u16 0 items=["Auto", "Limited", "Fixed"] ("Gate Range\nmode 2")
          }
          frame "f" {
            w592 = u16 2 items=["Auto", "Limited", "Fixed"] ("Gate Range\nmode 2")
          }
          frame "l" {
            w593 = u16 1 items=["Auto", "Limited", "Fixed"] ("Gate Range\nmode 2")
          }
        }
      }
      frame "gaterange" {
        (unwired) u8 11 items=["10fA  ", "100fA  ", "1nA  ", "10nA", "100nA", "1uA", "10uA", "100uA", "1mA", "10mA", "100mA", "1A"] ("Gate Range 2")
        n168 = Delete From Array(array=w613, index=0 ("Index")) -> (deleted portion=w603:string)  [unwired: 1 in, 1 out]
        n169 = Scan Value(string=w603, format string="") -> (value=w601:dbl)  [unwired: 1 in, 1 out]
        n170 = Logarithm Base 10(1:w601) -> (0:w600:dbl)
        n171 = Round To Nearest(number=w600) -> (nearest integer value=w599:dbl)
        n172 = Add(x=w599, y=11.0) -> (x+y=w597:dbl)
        n173 = To Unsigned Byte Integer(number=w597) -> (unsigned 8bit integer=w596:u8)
      }
      frame "drainrange" {
        (unwired) u8 11 items=["10fA  ", "100fA  ", "1nA  ", "10nA", "100nA", "1uA", "10uA", "100uA", "1mA", "10mA", "100mA", "1A"] ("Gate Range 2")
        n174 = Delete From Array(array=w634, index=0 ("Index")) -> (deleted portion=w625:string)  [unwired: 1 in, 1 out]
        n175 = Scan Value(string=w625, format string="") -> (value=w623:dbl)  [unwired: 1 in, 1 out]
        n176 = Logarithm Base 10(1:w623) -> (0:w622:dbl)
        n177 = Round To Nearest(number=w622) -> (nearest integer value=w621:dbl)
        n178 = Add(x=w621, y=11.0) -> (x+y=w619:dbl)
        n179 = To Unsigned Byte Integer(number=w619) -> (unsigned 8bit integer=w618:u8)
      }
      frame "drainrangemode" {
        n180 = Delete From Array(array=w648, index=0 ("Index")) -> (deleted portion=w649:string)  [unwired: 1 in, 1 out]
        n181 = case shown="\"f\"" w649 {
          tunnel: [w651 w652 w653] -> w638
          frame "a", Default {
            w651 = u16 0 items=["Auto", "Limited", "Fixed"] ("Gate Range\nmode 2")
          }
          frame "f" {
            w652 = u16 2 items=["Auto", "Limited", "Fixed"] ("Gate Range\nmode 2")
          }
          frame "l" {
            w653 = u16 1 items=["Auto", "Limited", "Fixed"] ("Gate Range\nmode 2")
          }
        }
      }
      frame "Error", Default {
      }
      frame "logfile" {
        n182 = Number To Decimal String(number=w668) -> (decimal integer string=w703:string)  [unwired: 1 in]
        n183 = Concatenate Strings(w702, "logfile" ("Substring"), w703, w666, ".txt" ("Substring")) -> (w700:string)
        n184 = String To Path(string=w700) -> (path=w673:path)
        n185 = Unbundle(w699) -> ("integration time"=w698:u32, "Short/Long integration time"=w697:dbl, "hold time (sec)"=w696:dbl, "delay time (sec)"=w695:dbl, "Step Time (0 disables)"=w694:dbl, "sweep method"=w693:u16, "Pulse period"=w692:dbl, "Base voltage"=w691:dbl, "Pulse width"=w690:dbl)
        n186 = Build Array(w698, w697, w696, w695, w694, w693, w692, w691, w690, w684, w685, w686, w687, w688, w689) -> (w677:dbl[])
        n187 = Insert Into Array(array=dbl[][] [] ("Input Array"), new element=w677) -> (w676:dbl[][])  [unwired: 2 in]
        n188 = call <vilib>:"compatOverwrite.vi"("overwrite (F)"=TRUE) -> ("overwrite?"=w671:T7)
        n189 = Open/Create/Replace File(file path (use dialog)=w673, error in=w675, operation (0:open)=w671) -> (refnum out=w681:refnum<file>, error out=w680:errorcluster)  [unwired: 3 in, 1 out]
        n190 = call <userlib>:"4155C Write array to file.vi"("Byte Stream File Refnum"=w681, "Header"=string[] ["Int Time", "Short/Long Itime", "Hold time", "Delay time", "Step time", "Sweep method", "Pulse period", "Base Voltage", "Pulse width", "Drain compliance", "Gate compliance", "Gate range mode", "Gate range", "S/D range mode", "S/D range"], "Data Array"=w676, "error in (no error)"=w680) -> ("dup refnum"=w683:refnum<file>, "error out"=w682:errorcluster)  [unwired: 1 in]
        n191 = Close File(refnum=w683, error in=w682) -> (error out=w674:errorcluster)  [unwired: 1 out]
      }
      frame "sample" {
        n192 = Number To Decimal String(number=w707) -> (decimal integer string=w755:string)  [unwired: 1 in]
        n193 = Fract/Exp String To Number(string=w752) -> (number=w713:dbl[])  [unwired: 3 in, 1 out]
        n194 = Concatenate Strings(w730, "-sample-" ("Substring"), w755, w705, ".txt" ("Substring")) -> (w753:string)
        n195 = String To Path(string=w753) -> (path=w734:path)
        n196 = Index Array(array=w713, index=0 ("Index")) -> (element=w750:dbl)
        n197 = Index Array(array=w713, index=2 ("Index")) -> (element=w746:dbl)
        n198 = Index Array(array=w713, index=3 ("Index")) -> (element=w715:dbl)
        n199 = Index Array(array=w713, index=4 ("Index")) -> (element=w712:dbl)
        n200 = call <userlib>:"4155C Config Sampling Measurements.vi"("Sampling interval"=w712, "Sample time"=w715, "Display on/off"=TRUE, "Timings"=w721, "Num Points"=w746, "error in (no error)"=w757, "Drain Compliance"=w756, "Gate Compliance"=w731, "VISA session"=w758) -> ("error out"=w759:errorcluster, "dup VISA resource name"=w760:refnum<visa-resource-name>)  [unwired: 1 in]
        n201 = Index Array(array=w713, index=1 ("Index")) -> (element=w747:dbl)
        n202 = call <userlib>:"4155C Take Sample.vi"("Emergency Stop"=w727, "error in (no error)"=w759, "Vd"=w747, "Vg"=w750, "VISA resource name in"=w760) -> ("error out"=w725:errorcluster, "Id"=w762:dbl[], "Ig"=w736:dbl[], "VISA Resource Name out"=w723:refnum<visa-resource-name>, "Is"=w761:dbl[], "Time"=w740:dbl[])  [unwired: 1 in]
        n203 = Insert Into Array(array=dbl[][] [] ("Input Array"), new element=w740) -> (w739:dbl[][])  [unwired: 2 in]
        n204 = Insert Into Array(array=w739, new element=w736) -> (w738:dbl[][])  [unwired: 2 in]
        n205 = Insert Into Array(array=w738, new element=w762) -> (w737:dbl[][])  [unwired: 2 in]
        n206 = VISA Write(VISA resource name=w723, write buffer=":DISP ON" ("write buffer (\"\")"), error in (no error)=w725) -> (VISA resource name out=w722:refnum<visa-resource-name>, error out=w724:errorcluster)  [unwired: 1 out]
        n207 = Insert Into Array(array=w737, new element=w761) -> (w729:dbl[][])  [unwired: 2 in]
        n208 = Transpose 2D Array(2D array=w729) -> (transposed array=w728:dbl[][])
        n209 = call <vilib>:"compatOverwrite.vi"("overwrite (F)"=TRUE) -> ("overwrite?"=w710:T7)
        n210 = Open/Create/Replace File(file path (use dialog)=w734, error in=w724, operation (0:open)=w710) -> (refnum out=w743:refnum<file>, error out=w742:errorcluster)  [unwired: 3 in, 1 out]
        n211 = call <userlib>:"4155C Write array to file.vi"("Byte Stream File Refnum"=w743, "Header"=string[] ["Time /s", "Ig /A", "Id /A", "Is /A"], "Data Array"=w728, "error in (no error)"=w742) -> ("dup refnum"=w745:refnum<file>, "error out"=w744:errorcluster)  [unwired: 1 in]
        n212 = Close File(refnum=w745, error in=w744) -> (error out=w732:errorcluster)  [unwired: 1 out]
      }
      frame "samplei" {
        n213 = Number To Decimal String(number=w764) -> (decimal integer string=w816:string)  [unwired: 1 in]
        n214 = Fract/Exp String To Number(string=w813) -> (number=w780:dbl[])  [unwired: 3 in, 1 out]
        n215 = Concatenate Strings(w795, "-samplei-" ("Substring"), w816, w763, ".txt" ("Substring")) -> (w814:string)
        n216 = String To Path(string=w814) -> (path=w798:path)
        n217 = Index Array(array=w780, index=4 ("Index")) -> (element=w774:dbl)
        n218 = Index Array(array=w780, index=3 ("Index")) -> (element=w775:dbl)
        n219 = Index Array(array=w780, index=1 ("Index")) -> (element=w777:dbl)
        n220 = Index Array(array=w780, index=0 ("Index")) -> (element=w778:dbl)
        n221 = Index Array(array=w780, index=2 ("Index")) -> (element=w776:dbl)
        n222 = call <userlib>:"4155C Config SamplingI Measurements.vi"("Sample time"=w776, "Display on/off"=TRUE, "Timings"=w787, "Num Points"=w777, "error in (no error)"=w818, "Sampling interval"=w775, "VISA session"=w819) -> ("error out"=w820:errorcluster, "dup VISA resource name"=w821:refnum<visa-resource-name>)  [unwired: 3 in]
        n223 = call <userlib>:"4155C Take SampleI.vi"("Emergency Stop"=w792, "error in (no error)"=w820, "Idg 2"=w778, "Vdg compliance 2"=w774, "VISA resource name in"=w821) -> ("error out"=w790:errorcluster, "Idg"=w823:dbl[], "Vdg"=w800:dbl[], "VISA Resource Name out"=w788:refnum<visa-resource-name>, "Is"=w822:dbl[], "Time"=w804:dbl[])  [unwired: 1 in]
        n224 = Insert Into Array(array=dbl[][] [] ("Input Array"), new element=w804) -> (w803:dbl[][])  [unwired: 2 in]
        n225 = Insert Into Array(array=w803, new element=w800) -> (w802:dbl[][])  [unwired: 2 in]
        n226 = Insert Into Array(array=w802, new element=w823) -> (w801:dbl[][])  [unwired: 2 in]
        n227 = VISA Write(VISA resource name=w788, write buffer=":DISP ON" ("write buffer (\"\")"), error in (no error)=w790) -> (VISA resource name out=w773:refnum<visa-resource-name>, error out=w789:errorcluster)  [unwired: 1 out]
        n228 = Insert Into Array(array=w801, new element=w822) -> (w794:dbl[][])  [unwired: 2 in]
        n229 = Transpose 2D Array(2D array=w794) -> (transposed array=w793:dbl[][])
        n230 = call <vilib>:"compatOverwrite.vi"("overwrite (F)"=TRUE) -> ("overwrite?"=w768:T7)
        n231 = Open/Create/Replace File(file path (use dialog)=w798, error in=w789, operation (0:open)=w768) -> (refnum out=w807:refnum<file>, error out=w806:errorcluster)  [unwired: 3 in, 1 out]
        n232 = call <userlib>:"4155C Write array to file.vi"("Byte Stream File Refnum"=w807, "Header"=string[] ["Time /s", "Vdg /V", "Idg /A", "Is /A"], "Data Array"=w793, "error in (no error)"=w806) -> ("dup refnum"=w809:refnum<file>, "error out"=w808:errorcluster)  [unwired: 1 in]
        n233 = Close File(refnum=w809, error in=w808) -> (error out=w771:errorcluster)  [unwired: 1 out]
        n234 = VISA Write(VISA resource name=w773, write buffer=";:PAGE:SCON:STAN OFF;:PAGE:CHAN:VSU2:DIS;" ("write buffer (\"\")"), error in (no error)=w771) -> (VISA resource name out=w769:refnum<visa-resource-name>, error out=w770:errorcluster)  [unwired: 1 out]
      }
      frame "#" {
        n235 = VISA Write(VISA resource name=w830, write buffer=":DISP ON" ("write buffer (\"\")"), error in (no error)=w829) -> (VISA resource name out=w828:refnum<visa-resource-name>, error out=w827:errorcluster)  [unwired: 1 out]
      }
      frame "stressV" {
        n236 = Number To Decimal String(number=w840) -> (decimal integer string=w881:string)  [unwired: 1 in]
        n237 = Fract/Exp String To Number(string=w878) -> (number=w851:dbl[])  [unwired: 3 in, 1 out]
        n238 = Concatenate Strings(w865, "-stressV-" ("Substring"), w881, w839, ".txt" ("Substring")) -> (w879:string)
        n239 = String To Path(string=w879) -> (path=w869:path)
        n240 = Index Array(array=w851, index=3 ("Index")) -> (element=w848:dbl)
        n241 = Index Array(array=w851, index=1 ("Index")) -> (element=w846:dbl)
        n242 = Index Array(array=w851, index=0 ("Index")) -> (element=w845:dbl)
        n243 = Index Array(array=w851, index=4 ("Index")) -> (element=w850:dbl)
        n244 = Index Array(array=w851, index=2 ("Index")) -> (element=w847:dbl)
        n245 = call <userlib>:"4155C Config V Stress.vi"("VISA session"=w884, "ID compliance"=w848, "VD"=w846, "VG"=w845, "IG compliance"=w847, "error in (no error)"=w883, "Display on/off"=TRUE) -> ("dup VISA resource name"=w886:refnum<visa-resource-name>, "error out"=w885:errorcluster)
        n246 = call <userlib>:"4155C Apply Stress.vi"("error in (no error)"=w885, "Duration"=w850, "Emergency Stop"=w864, "VISA resource name in"=w886) -> ("error out"=w862:errorcluster, "VISA Resource Name out"=w860:refnum<visa-resource-name>)
        n247 = VISA Write(VISA resource name=w860, write buffer=":DISP ON" ("write buffer (\"\")"), error in (no error)=w862) -> (VISA resource name out=w859:refnum<visa-resource-name>, error out=w861:errorcluster)  [unwired: 1 out]
        n248 = call <vilib>:"compatOverwrite.vi"("overwrite (F)"=TRUE) -> ("overwrite?"=w844:T7)
        n249 = Open/Create/Replace File(file path (use dialog)=w869, error in=w861, operation (0:open)=w844) -> (refnum out=w872:refnum<file>, error out=w871:errorcluster)  [unwired: 3 in, 1 out]
        n250 = call <userlib>:"4155C Write array to file.vi"("Byte Stream File Refnum"=w872, "Header"=string[] ["V stress completed successfully", ""], "error in (no error)"=w871) -> ("dup refnum"=w874:refnum<file>, "error out"=w873:errorcluster)  [unwired: 2 in]
        n251 = Close File(refnum=w874, error in=w873) -> (error out=w867:errorcluster)  [unwired: 1 out]
      }
      frame "stressI" {
        n252 = Number To Decimal String(number=w888) -> (decimal integer string=w925:string)  [unwired: 1 in]
        n253 = Fract/Exp String To Number(string=w922) -> (number=w897:dbl[])  [unwired: 3 in, 1 out]
        n254 = Concatenate Strings(w909, "-stressI-" ("Substring"), w925, w887, ".txt" ("Substring")) -> (w923:string)
        n255 = String To Path(string=w923) -> (path=w913:path)
        n256 = Index Array(array=w897, index=1 ("Index")) -> (element=w893:dbl)
        n257 = Index Array(array=w897, index=0 ("Index")) -> (element=w894:dbl)
        n258 = call <userlib>:"4155C Config I Stress.vi"("VISA session"=w928, "IDG"=w894, "VDG compliance"=w893, "error in (no error)"=w927, "Display on/off"=TRUE) -> ("dup VISA resource name"=w930:refnum<visa-resource-name>, "error out"=w929:errorcluster)
        n259 = Index Array(array=w897, index=2 ("Index")) -> (element=w895:dbl)
        n260 = call <userlib>:"4155C Apply Stress.vi"("error in (no error)"=w929, "Duration"=w895, "Emergency Stop"=w908, "VISA resource name in"=w930) -> ("error out"=w906:errorcluster, "VISA Resource Name out"=w904:refnum<visa-resource-name>)
        n261 = VISA Write(VISA resource name=w904, write buffer=":DISP ON" ("write buffer (\"\")"), error in (no error)=w906) -> (VISA resource name out=w903:refnum<visa-resource-name>, error out=w905:errorcluster)  [unwired: 1 out]
        n262 = call <vilib>:"compatOverwrite.vi"("overwrite (F)"=TRUE) -> ("overwrite?"=w892:T7)
        n263 = Open/Create/Replace File(file path (use dialog)=w913, error in=w905, operation (0:open)=w892) -> (refnum out=w916:refnum<file>, error out=w915:errorcluster)  [unwired: 3 in, 1 out]
        n264 = call <userlib>:"4155C Write array to file.vi"("Byte Stream File Refnum"=w916, "Header"=string[] ["I stress completed successfully", ""], "error in (no error)"=w915) -> ("dup refnum"=w918:refnum<file>, "error out"=w917:errorcluster)  [unwired: 2 in]
        n265 = Close File(refnum=w918, error in=w917) -> (error out=w911:errorcluster)  [unwired: 1 out]
      }
      frame "vsu2pulse" {
        n266 = Number To Decimal String(number=w932) -> (decimal integer string=w967:string)  [unwired: 1 in]
        n267 = Fract/Exp String To Number(string=w964) -> (number=w940:dbl[])  [unwired: 3 in, 1 out]
        n268 = Concatenate Strings(w952, "-vsu2-" ("Substring"), w967, w931, ".txt" ("Substring")) -> (w965:string)
        n269 = String To Path(string=w965) -> (path=w956:path)
        n270 = Index Array(array=w940, index=1 ("Index")) -> (element=w939:dbl)
        n271 = Index Array(array=w940, index=0 ("Index")) -> (element=w937:dbl)
        n272 = call <userlib>:"4155C Config VSU2 Stress.vi"("error in (no error)"=w969, "VSU2"=w937, "Display on/off"=TRUE, "VISA session"=w970) -> ("error out"=w971:errorcluster, "dup VISA resource name"=w972:refnum<visa-resource-name>)
        n273 = call <userlib>:"4155C Apply Stress.vi"("error in (no error)"=w971, "Duration"=w939, "Emergency Stop"=w951, "VISA resource name in"=w972) -> ("error out"=w949:errorcluster, "VISA Resource Name out"=w947:refnum<visa-resource-name>)
        n274 = VISA Write(VISA resource name=w947, write buffer=":DISP ON" ("write buffer (\"\")"), error in (no error)=w949) -> (VISA resource name out=w946:refnum<visa-resource-name>, error out=w948:errorcluster)  [unwired: 1 out]
        n275 = call <vilib>:"compatOverwrite.vi"("overwrite (F)"=TRUE) -> ("overwrite?"=w936:T7)
        n276 = Open/Create/Replace File(file path (use dialog)=w956, error in=w948, operation (0:open)=w936) -> (refnum out=w959:refnum<file>, error out=w958:errorcluster)  [unwired: 3 in, 1 out]
        n277 = call <userlib>:"4155C Write array to file.vi"("Byte Stream File Refnum"=w959, "Header"=string[] ["VSU2 pulse completed successfully", ""], "error in (no error)"=w958) -> ("dup refnum"=w961:refnum<file>, "error out"=w960:errorcluster)  [unwired: 2 in]
        n278 = Close File(refnum=w961, error in=w960) -> (error out=w954:errorcluster)  [unwired: 1 out]
      }
      frame "sample-fpp" {
        w985 = string[] ["Time /s", "Id VgVd /A", "Ig VgVd /A", "Vp1 VgVd /V", "Vp2 VgVd /V"] ("Header")
        w989 = "%d" ("format string")
        n279 = Number To Decimal String(number=w974) -> (decimal integer string=w1037:string)  [unwired: 1 in]
        n280 = Fract/Exp String To Number(string=w1034) -> (number=w1022:dbl[])  [unwired: 3 in, 1 out]
        n281 = Concatenate Strings(w1028, "-samplefpp-" ("Substring"), w1037, w973, ".txt" ("Substring")) -> (w1035:string)
        n282 = String To Path(string=w1035) -> (path=w997:path)
        n283 = Index Array(array=w1022, index=0 ("Index")) -> (element=w983:dbl)
        n284 = Index Array(array=w1022, index=1 ("Index")) -> (element=w982:dbl)
        n285 = Index Array(array=w1022, index=2 ("Index")) -> (element=w1030:dbl)
        n286 = Index Array(array=w1022, index=3 ("Index")) -> (element=w1020:dbl)
        n287 = call <userlib>:"4155C Config Sampling Measurements FPP.vi"("VISA session"=w1040, "Num Points"=w1030, "Vg"=w983, "Display on/off"=TRUE, "Gate Compliance"=w1029, "Drain Compliance"=w1038, "Standby"="Standby", "error in (no error)"=w1039, "Timings"=w1027, "Vd"=w982, "Sample time"=w1020) -> ("dup VISA resource name"=w999:refnum<visa-resource-name>, "error out"=w998:errorcluster)  [unwired: 3 in]
        n288 = Number To Decimal String(number=w983) -> (decimal integer string=w1009:string)  [unwired: 1 in]
        n289 = call <userlib>:"4155C Take Sample FPP.vi"("VISA resource name in"=w999, "error in (no error)"=w998, "Emergency Stop"=w1000) -> ("Time"=w1004:dbl[], "Vp1"=w1014:dbl[], "VISA Resource Name out"=w980:refnum<visa-resource-name>, "Ig"=w1002:dbl[], "Id"=w1003:dbl[], "Vp2"=w1012:dbl[], "error out"=w1001:errorcluster)  [unwired: 10 in]
        n290 = Insert Into Array(array=dbl[][] [] ("Input Array"), new element=w1004) -> (w1018:dbl[][])  [unwired: 2 in]
        n291 = Number To Decimal String(number=w982) -> (decimal integer string=w1007:string)  [unwired: 1 in]
        n292 = Insert Into Array(array=w1018, new element=w1003) -> (w1017:dbl[][])  [unwired: 2 in]
        n293 = Concatenate Strings("(Vg = " ("Substring"), w1009, "V, Vd = " ("Substring"), w1007, "V)" ("Substring")) -> (w1005:string)
        n294 = Insert Into Array(array=w1017, new element=w1002) -> (w1016:dbl[][])  [unwired: 2 in]
        n295 = Insert Into Array(array=w1016, new element=w1014) -> (w1013:dbl[][])  [unwired: 2 in]
        n296 = Insert Into Array(array=w1013, new element=w1012) -> (w981:dbl[][])  [unwired: 2 in]
        n297 = call <vilib>:"compatOverwrite.vi"("overwrite (F)"=TRUE) -> ("overwrite?"=w978:T7)
        n298 = Open/Create/Replace File(file path (use dialog)=w997, error in=w1001, operation (0:open)=w978) -> (refnum out=w994:refnum<file>, error out=w995:errorcluster)  [unwired: 3 in, 1 out]
        n299 = Array To Spreadsheet String(array=w985, 3:w989) -> (spreadsheet string=w991:string)  [unwired: 1 in]
        n300 = Transpose 2D Array(2D array=w981) -> (transposed array=w1011:dbl[][])
        n301 = Search and Replace String(replace all?=TRUE ("replace all? (F)"), input string=w991, search string="VgVd", replace string=w1005) -> (result string=w987:string)  [unwired: 4 in, 3 out]
        n302 = Spreadsheet String To Array(format string=w989, spreadsheet string=w987, array type (2D Dbl)=w985) -> (array=w986:string[])  [unwired: 1 in]
        n303 = call <userlib>:"4155C Write array to file.vi"("Byte Stream File Refnum"=w994, "Header"=w986, "Data Array"=w1011, "error in (no error)"=w995) -> ("dup refnum"=w992:refnum<file>, "error out"=w993:errorcluster)  [unwired: 1 in]
        n304 = Close File(refnum=w992, error in=w993) -> (error out=w979:errorcluster)  [unwired: 1 out]
      }
      frame "resample-fpp" {
        w1055 = string[] ["Time /s", "Id VgVd /A", "Ig VgVd /A", "Vp1 VgVd /V", "Vp2 VgVd /V"] ("Header")
        w1059 = "%d" ("format string")
        n305 = Number To Decimal String(number=w1041) -> (decimal integer string=w1099:string)  [unwired: 1 in]
        n306 = Fract/Exp String To Number(string=w1096) -> (number=w1048:dbl[])  [unwired: 3 in, 1 out]
        n307 = Concatenate Strings(w1092, "-resamplefpp-" ("Substring"), w1099, w1042, ".txt" ("Substring")) -> (w1097:string)
        n308 = String To Path(string=w1097) -> (path=w1067:path)
        n309 = Index Array(array=w1048, index=0 ("Index")) -> (element=w1054:dbl)
        n310 = Index Array(array=w1048, index=1 ("Index")) -> (element=w1053:dbl)
        n311 = Number To Decimal String(number=w1054) -> (decimal integer string=w1077:string)  [unwired: 1 in]
        n312 = call <userlib>:"4155C Take Sample FPP.vi"("VISA resource name in"=w1050, "error in (no error)"=w1049, "Emergency Stop"=w1068) -> ("Time"=w1072:dbl[], "Vp1"=w1082:dbl[], "VISA Resource Name out"=w1052:refnum<visa-resource-name>, "Ig"=w1070:dbl[], "Id"=w1071:dbl[], "Vp2"=w1080:dbl[], "error out"=w1069:errorcluster)  [unwired: 10 in]
        n313 = Insert Into Array(array=dbl[][] [] ("Input Array"), new element=w1072) -> (w1086:dbl[][])  [unwired: 2 in]
        n314 = Number To Decimal String(number=w1053) -> (decimal integer string=w1075:string)  [unwired: 1 in]
        n315 = Insert Into Array(array=w1086, new element=w1071) -> (w1085:dbl[][])  [unwired: 2 in]
        n316 = Concatenate Strings("(Vg = " ("Substring"), w1077, "V, Vd = " ("Substring"), w1075, "V)" ("Substring")) -> (w1073:string)
        n317 = Insert Into Array(array=w1085, new element=w1070) -> (w1084:dbl[][])  [unwired: 2 in]
        n318 = Insert Into Array(array=w1084, new element=w1082) -> (w1081:dbl[][])  [unwired: 2 in]
        n319 = Insert Into Array(array=w1081, new element=w1080) -> (w1047:dbl[][])  [unwired: 2 in]
        n320 = call <vilib>:"compatOverwrite.vi"("overwrite (F)"=TRUE) -> ("overwrite?"=w1046:T7)
        n321 = Open/Create/Replace File(file path (use dialog)=w1067, error in=w1069, operation (0:open)=w1046) -> (refnum out=w1064:refnum<file>, error out=w1065:errorcluster)  [unwired: 3 in, 1 out]
        n322 = Array To Spreadsheet String(array=w1055, 3:w1059) -> (spreadsheet string=w1061:string)  [unwired: 1 in]
        n323 = Transpose 2D Array(2D array=w1047) -> (transposed array=w1079:dbl[][])
        n324 = Search and Replace String(replace all?=TRUE ("replace all? (F)"), input string=w1061, search string="VgVd", replace string=w1073) -> (result string=w1057:string)  [unwired: 4 in, 3 out]
        n325 = Spreadsheet String To Array(format string=w1059, spreadsheet string=w1057, array type (2D Dbl)=w1055) -> (array=w1056:string[])  [unwired: 1 in]
        n326 = call <userlib>:"4155C Write array to file.vi"("Byte Stream File Refnum"=w1064, "Header"=w1056, "Data Array"=w1079, "error in (no error)"=w1065) -> ("dup refnum"=w1062:refnum<file>, "error out"=w1063:errorcluster)  [unwired: 1 in]
        n327 = Close File(refnum=w1062, error in=w1063) -> (error out=w1051:errorcluster)  [unwired: 1 out]
      }
      frame "serial" {
        n328 = Index Array(array=w1102, index=0 ("Index")) -> (element=w1101:string)
        n329 = call <userlib>:"Serial write and read v0.2.vi"("Pump No"="Pump No", "Termination char\n(0xA = '\\n' = LF)\n(0xD = '\\r' = CR)"="Termination char\n(0xA = '\\n' = LF)\n(0xD = '\\r' = CR)", "Enable Termination\nChar (T)"="Enable Termination\nChar (T)", "parity"="parity", "stop bits"="stop bits", "string to write"=w1101, "flow control"="flow control", "bytes to read"="bytes to read", "Serial Settings:Serial End Mode for Reads"="Serial Settings:Serial End Mode for Reads", "Timeout (ms)"="Timeout (ms)", "error in (no error)"=w1107, "VISA resource name"="VISA resource name", "baud rate"="baud rate", "data bits"="data bits") -> ("read string"=→"Serial output":string, "error out"=w1106:errorcluster)
      }
    }
    n330 = Empty String/Path?(string/path=w50) -> (empty?=w85:bool)
    n331 = Not(x=w85) -> (.not. x?=w84:bool)
  }
  "error out" <- w2
